vi "main.vi"() -> ()   [LabVIEW 2019]
uses:
  Globals.vi
  <vilib>/Utility/config.llb/NI_LVConfig.lvlib
panel:
  in  "sorted":bool
  in  "compare":bool
  in  "Presets":bool
  in  "Data":u16(ring) items=["cumulative cases", "new cases per day", "cumulative deaths", "new deaths per day"]
  in  "Compare with":u16(ring) items=["Don't compare", "Afghanistan", "Albania", "Algeria", "Andorra", "Angola", "Antigua and Barbuda", "Argentina", "Armenia", "Australia, Australian Capital Territory", "Australia, New South Wales", "Australia, Northern Territory", "Australia, Queensland", "Australia, South Australia", "Australia, Tasmania", "Australia, Victoria", "Australia, Western Australia", "Austria", "Azerbaijan", "Bahamas", "Bahrain", "Bangladesh", "Barbados", "Belarus", "Belgium", "Benin", "Bhutan", "Bolivia", "Bosnia and Herzegovina", "Brazil", "Brunei", "Bulgaria", "Burkina Faso", "Cabo Verde", "Cambodia", "Cameroon", "Canada, Alberta", "Canada, British Columbia", "Canada, Grand Princess", "Canada, Manitoba", "Canada, New Brunswick", "Canada, Newfoundland and Labrador", "Canada, Nova Scotia", "Canada, Ontario", "Canada, Prince Edward Island", "Canada, Quebec", "Canada, Saskatchewan", "Central African Republic", "Chad", "Chile", "China, Anhui", "China, Beijing", "China, Chongqing", "China, Fujian", "China, Gansu", "China, Guangdong", "China, Guangxi", "China, Guizhou", "China, Hainan", "China, Hebei", "China, Heilongjiang", "China, Henan", "China, Hong Kong", "China, Hubei", "China, Hunan", "China, Inner Mongolia", "China, Jiangsu", "China, Jiangxi", "China, Jilin", "China, Liaoning", "China, Macau", "China, Ningxia", "China, Qinghai", "China, Shaanxi", "China, Shandong", "China, Shanghai", "China, Shanxi", "China, Sichuan", "China, Tianjin", "China, Tibet", "China, Xinjiang", "China, Yunnan", "China, Zhejiang", "Colombia", "Congo (Brazzaville)", "Congo (Kinshasa)", "Costa Rica", "Cote d'Ivoire", "Croatia", "Diamond Princess", "Cuba", "Cyprus", "Czechia", "Denmark, Faroe Islands", "Denmark, Greenland", "Denmark", "Djibouti", "Dominican Republic", "Ecuador", "Egypt", "El Salvador", "Equatorial Guinea", "Eritrea", "Estonia", "Eswatini", "Ethiopia", "Fiji", "Finland", "France, French Guiana", "France, French Polynesia", "France, Guadeloupe", "France, Mayotte", "France, New Caledonia", "France, Reunion", "France, Saint Barthelemy", "France, St Martin", "France, Martinique", "France", "Gabon", "Gambia", "Georgia", "Germany", "Ghana", "Greece", "Guatemala", "Guinea", "Guyana", "Haiti", "Holy See", "Honduras", "Hungary", "Iceland", "India", "Indonesia", "Iran", "Iraq", "Ireland", "Israel", "Italy", "Jamaica", "Japan", "Jordan", "Kazakhstan", "Kenya", "Korea South", "Kuwait", "Kyrgyzstan", "Latvia", "Lebanon", "Liberia", "Liechtenstein", "Lithuania", "Luxembourg", "Madagascar", "Malaysia", "Maldives", "Malta", "Mauritania", "Mauritius", "Mexico", "Moldova", "Monaco", "Mongolia", "Montenegro", "Morocco", "Namibia", "Nepal", "Netherlands, Aruba", "Netherlands, Curacao", "Netherlands, Sint Maarten", "Netherlands", "New Zealand", "Nicaragua", "Niger", "Nigeria", "North Macedonia", "Norway", "Oman", "Pakistan", "Panama", "Papua New Guinea", "Paraguay", "Peru", "Philippines", "Poland", "Portugal", "Qatar", "Romania", "Russia", "Rwanda", "Saint Lucia", "Saint Vincent and the Grenadines", "San Marino", "Saudi Arabia", "Senegal", "Serbia", "Seychelles", "Singapore", "Slovakia", "Slovenia", "Somalia", "South Africa", "Spain", "Sri Lanka", "Sudan", "Suriname", "Sweden", "Switzerland", "Taiwan*", "Tanzania", "Thailand", "Togo", "Trinidad and Tobago", "Tunisia", "Turkey", "Uganda", "Ukraine", "United Arab Emirates", "United Kingdom, Bermuda", "United Kingdom, Cayman Islands", "United Kingdom, Channel Islands", "United Kingdom, Gibraltar", "United Kingdom, Isle of Man", "United Kingdom, Montserrat", "United Kingdom", "Uruguay", "US", "Uzbekistan", "Venezuela", "Vietnam", "Zambia", "Zimbabwe", "Canada, Diamond Princess", "Dominica", "Grenada", "Mozambique", "Syria", "Timor-Leste", "Belize", "Laos", "Libya", "West Bank and Gaza", "Guinea-Bissau", "Mali", "Saint Kitts and Nevis", "Canada, Northwest Territories", "Canada, Yukon", "Kosovo", "Burma", "United Kingdom, Anguilla", "United Kingdom, British Virgin Islands", "United Kingdom, Turks and Caicos Islands", "MS Zaandam", "Botswana", "Burundi", "Sierra Leone", "Netherlands, \"Bonaire Sint Eustatius and Saba\"", "Malawi", "United Kingdom, Falkland Islands (Malvinas)", "France, Saint Pierre and Miquelon", "South Sudan", "Western Sahara", "Sao Tome and Principe", "Yemen", "Comoros", "Tajikistan", "Lesotho", "Australia", "Western Europe", "Latin America", "Africa", "China", "US and Canada", "US - Northeast", "US - Midwest", "US - South", "US - West", "Scandinavia (excl Sweden)", "Global", "South Asia", "South East Asia", "East Asia", "Eastern Europe and Russia", "Middle East", "Central Asia", "American Samoa", "Guam", "Northern Mariana Islands", "Puerto Rico", "Virgin Islands", "Alabama", "Alaska", "Arizona", "Arkansas", "California", "Colorado", "Connecticut", "Delaware", "Florida", "Georgia", "Hawaii", "Idaho", "Illinois", "Indiana", "Iowa", "Kansas", "Kentucky", "Louisiana", "Maine", "Maryland", "Massachusetts", "Michigan", "Minnesota", "Mississippi", "Missouri", "Montana", "Nebraska", "Nevada", "New Hampshire", "New Jersey", "New Mexico", "New York", "North Carolina", "North Dakota", "Ohio", "Oklahoma", "Oregon", "Pennsylvania", "Rhode Island", "South Carolina", "South Dakota", "Tennessee", "Texas", "Utah", "Vermont", "Virginia", "Washington", "West Virginia", "Wisconsin", "Wyoming", "SA, EC", "SA, FS", "SA, GP", "SA, KZN", "SA, LP", "SA, MP", "SA, NC", "SA, NW", "SA, WC"]
  in  "Country":u16(ring) items=["Afghanistan", "Albania", "Algeria", "Andorra", "Angola", "Antigua and Barbuda", "Argentina", "Armenia", "Australia, Australian Capital Territory", "Australia, New South Wales", "Australia, Northern Territory", "Australia, Queensland", "Australia, South Australia", "Australia, Tasmania", "Australia, Victoria", "Australia, Western Australia", "Austria", "Azerbaijan", "Bahamas", "Bahrain", "Bangladesh", "Barbados", "Belarus", "Belgium", "Benin", "Bhutan", "Bolivia", "Bosnia and Herzegovina", "Brazil", "Brunei", "Bulgaria", "Burkina Faso", "Cabo Verde", "Cambodia", "Cameroon", "Canada, Alberta", "Canada, British Columbia", "Canada, Grand Princess", "Canada, Manitoba", "Canada, New Brunswick", "Canada, Newfoundland and Labrador", "Canada, Nova Scotia", "Canada, Ontario", "Canada, Prince Edward Island", "Canada, Quebec", "Canada, Saskatchewan", "Central African Republic", "Chad", "Chile", "China, Anhui", "China, Beijing", "China, Chongqing", "China, Fujian", "China, Gansu", "China, Guangdong", "China, Guangxi", "China, Guizhou", "China, Hainan", "China, Hebei", "China, Heilongjiang", "China, Henan", "China, Hong Kong", "China, Hubei", "China, Hunan", "China, Inner Mongolia", "China, Jiangsu", "China, Jiangxi", "China, Jilin", "China, Liaoning", "China, Macau", "China, Ningxia", "China, Qinghai", "China, Shaanxi", "China, Shandong", "China, Shanghai", "China, Shanxi", "China, Sichuan", "China, Tianjin", "China, Tibet", "China, Xinjiang", "China, Yunnan", "China, Zhejiang", "Colombia", "Congo (Brazzaville)", "Congo (Kinshasa)", "Costa Rica", "Cote d'Ivoire", "Croatia", "Diamond Princess", "Cuba", "Cyprus", "Czechia", "Denmark, Faroe Islands", "Denmark, Greenland", "Denmark", "Djibouti", "Dominican Republic", "Ecuador", "Egypt", "El Salvador", "Equatorial Guinea", "Eritrea", "Estonia", "Eswatini", "Ethiopia", "Fiji", "Finland", "France, French Guiana", "France, French Polynesia", "France, Guadeloupe", "France, Mayotte", "France, New Caledonia", "France, Reunion", "France, Saint Barthelemy", "France, St Martin", "France, Martinique", "France", "Gabon", "Gambia", "Georgia", "Germany", "Ghana", "Greece", "Guatemala", "Guinea", "Guyana", "Haiti", "Holy See", "Honduras", "Hungary", "Iceland", "India", "Indonesia", "Iran", "Iraq", "Ireland", "Israel", "Italy", "Jamaica", "Japan", "Jordan", "Kazakhstan", "Kenya", "Korea South", "Kuwait", "Kyrgyzstan", "Latvia", "Lebanon", "Liberia", "Liechtenstein", "Lithuania", "Luxembourg", "Madagascar", "Malaysia", "Maldives", "Malta", "Mauritania", "Mauritius", "Mexico", "Moldova", "Monaco", "Mongolia", "Montenegro", "Morocco", "Namibia", "Nepal", "Netherlands, Aruba", "Netherlands, Curacao", "Netherlands, Sint Maarten", "Netherlands", "New Zealand", "Nicaragua", "Niger", "Nigeria", "North Macedonia", "Norway", "Oman", "Pakistan", "Panama", "Papua New Guinea", "Paraguay", "Peru", "Philippines", "Poland", "Portugal", "Qatar", "Romania", "Russia", "Rwanda", "Saint Lucia", "Saint Vincent and the Grenadines", "San Marino", "Saudi Arabia", "Senegal", "Serbia", "Seychelles", "Singapore", "Slovakia", "Slovenia", "Somalia", "South Africa", "Spain", "Sri Lanka", "Sudan", "Suriname", "Sweden", "Switzerland", "Taiwan*", "Tanzania", "Thailand", "Togo", "Trinidad and Tobago", "Tunisia", "Turkey", "Uganda", "Ukraine", "United Arab Emirates", "United Kingdom, Bermuda", "United Kingdom, Cayman Islands", "United Kingdom, Channel Islands", "United Kingdom, Gibraltar", "United Kingdom, Isle of Man", "United Kingdom, Montserrat", "United Kingdom", "Uruguay", "US", "Uzbekistan", "Venezuela", "Vietnam", "Zambia", "Zimbabwe", "Canada, Diamond Princess", "Dominica", "Grenada", "Mozambique", "Syria", "Timor-Leste", "Belize", "Laos", "Libya", "West Bank and Gaza", "Guinea-Bissau", "Mali", "Saint Kitts and Nevis", "Canada, Northwest Territories", "Canada, Yukon", "Kosovo", "Burma", "United Kingdom, Anguilla", "United Kingdom, British Virgin Islands", "United Kingdom, Turks and Caicos Islands", "MS Zaandam", "Botswana", "Burundi", "Sierra Leone", "Netherlands, \"Bonaire Sint Eustatius and Saba\"", "Malawi", "United Kingdom, Falkland Islands (Malvinas)", "France, Saint Pierre and Miquelon", "South Sudan", "Western Sahara", "Sao Tome and Principe", "Yemen", "Comoros", "Tajikistan", "Lesotho", "Australia", "Western Europe", "Latin America", "Africa", "China", "US and Canada", "US - Northeast", "US - Midwest", "US - South", "US - West", "Scandinavia (excl Sweden)", "Global", "South Asia", "South East Asia", "East Asia", "Eastern Europe and Russia", "Middle East", "Central Asia", "American Samoa", "Guam", "Northern Mariana Islands", "Puerto Rico", "Virgin Islands", "Alabama", "Alaska", "Arizona", "Arkansas", "California", "Colorado", "Connecticut", "Delaware", "Florida", "Georgia", "Hawaii", "Idaho", "Illinois", "Indiana", "Iowa", "Kansas", "Kentucky", "Louisiana", "Maine", "Maryland", "Massachusetts", "Michigan", "Minnesota", "Mississippi", "Missouri", "Montana", "Nebraska", "Nevada", "New Hampshire", "New Jersey", "New Mexico", "New York", "North Carolina", "North Dakota", "Ohio", "Oklahoma", "Oregon", "Pennsylvania", "Rhode Island", "South Carolina", "South Dakota", "Tennessee", "Texas", "Utah", "Vermont", "Virginia", "Washington", "West Virginia", "Wisconsin", "Wyoming", "SA, EC", "SA, FS", "SA, GP", "SA, KZN", "SA, LP", "SA, MP", "SA, NC", "SA, NW", "SA, WC"]
  out "Version":u32
  in  "abs or rel":enum32{"Absolute", "Relative"}(tab)
  out "XY Graph":cluster{timestamp[], "deaths":dbl[]}[](graph)
  out "relative graph":cluster{"days":i32[], "deaths":dbl[]}[](graph)
  in  "calculate":bool
  in  "Days":u16=7
  in  "Moving average":bool
  in  "Y-axis normalised":bool
  in  "Y-axis absolute":bool caption="Y-axis"
  in  "Curve 2":enum16{"Exponential", "Logarithm", "No curve"}(ring)
  in  "Curve 1":enum16{"Exponential", "Logarithm", "No curve"}(ring)
  in  "X-axis relative":bool
  in  "X-axis absolute":bool caption="X-axis"
  in  "Curve fit cursors":bool
  in  "Curve fit all data":bool
  in  "Logarithmic":bool
  in  "threshold cases":u32=1
  in  "stop":bool
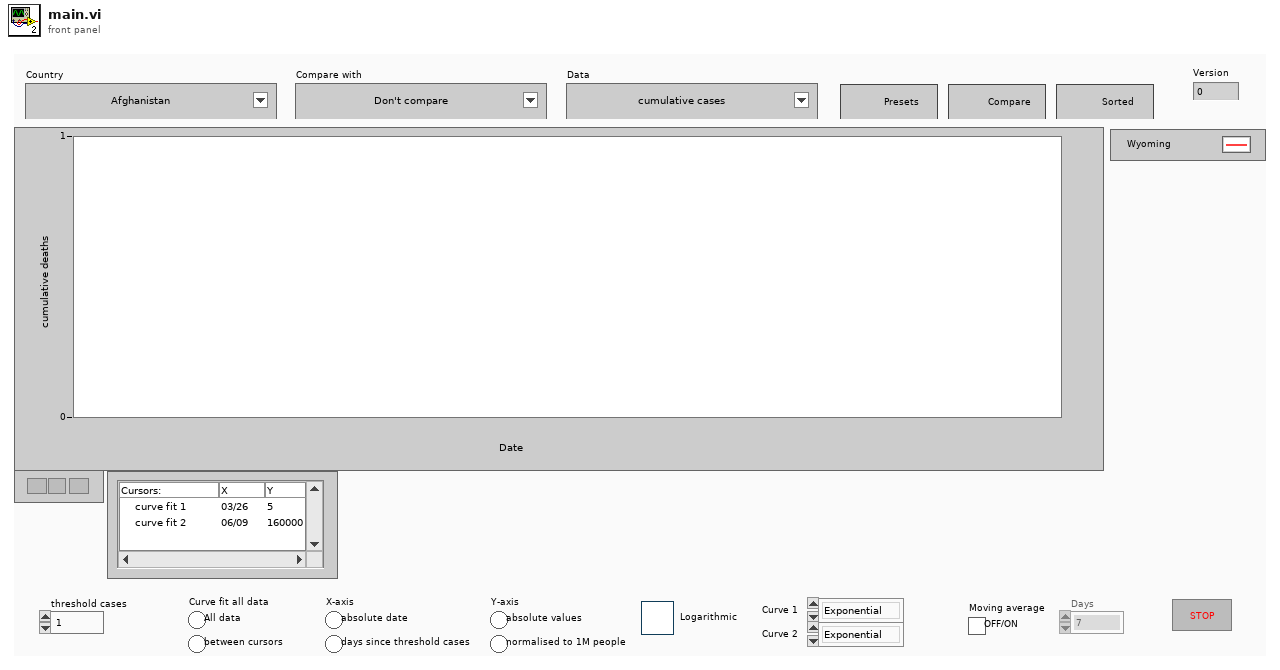
[diagram p1: front panel]
types:
  T1 = enum8{"Enabled", "Disabled", "Disabled and Grayed Out"}
  T2 = cluster{"country 1":cluster{"amplitude":dbl, "damping":dbl, "offset":dbl, "new cases per day":i32[], "days":i32[], "cumulative cases":i32[], "first case date":timestamp, "deaths":i32[], "new deaths per day":i32[]}, "country 2":cluster{"amplitude":dbl, "damping":dbl, "offset":dbl, "new cases per day":i32[], "days":i32[], "cumulative cases":i32[], "deaths":i32[], "first case date":timestamp, "new deaths per day":i32[]}, "Update plot names":refnum<user-event>}
  T3 = cluster{"cumulative deaths":i32[][], "deaths per day":i32[][], "case per day":i32[][], "cumulative cases":i32[][]}
  T4 = typedef "NI_LVConfig.lvlib/Config Data RefNum.ctl" = refnum<k1>
  T5 = cluster{"days":i32[], "new deaths per day":i32[]}
  T6 = cluster{"Country 1 index":i32, "Country 2 index":i32, "countries":string[], "Data":u16, "Curve fit all data":bool, "Curve 1 type":enum16{"Exponential", "Logarithm", "No curve"}, "Curve 2 type":enum16{"Exponential", "Logarithm", "No curve"}, "absolute?":bool, "cursor 1 ":dbl, "cursor 2 ":dbl, "threshold cases":u32}
  T7 = typedef "LVCursorListTypeDef.ctl" = cluster{"Name":string, "Color":u32, "Style":u8, "Point Style":u8, "Name Visible":bool, "Allow Drag":bool, "Cursor Mode":u32, "Plot":i32, "Index":i32, "Position":cluster{"X":dbl, "Y":dbl}, "X Scale":u32, "Y Scale":u32, "Watch Plots":i32[], "Watch All Plots":bool, "Plot Area":i32, "Label Offset":cluster{"X":dbl, "Y":dbl}}[]
  T8 = cluster{"Name":string, "Color":u32, "Style":u8, "Point Style":u8, "Name Visible":bool, "Allow Drag":bool, "Cursor Mode":u32, "Plot":i32, "Index":i32, "Position":cluster{"X":dbl, "Y":dbl}, "X Scale":u32, "Y Scale":u32, "Watch Plots":i32[], "Watch All Plots":bool, "Plot Area":i32, "Label Offset":cluster{"X":dbl, "Y":dbl}}
  T9 = cluster{"days":i32[], "moving average array":dbl[]}
  T10 = cluster{"days":i32[], "moving average array":dbl[]}[]
  T11 = cluster{timestamp[], "moving average array":dbl[]}
  T12 = cluster{timestamp[], "moving average array":dbl[]}[]
  T13 = cluster{"Name":string, "Color":u32, "Style":u8, "Point Style":u8, "Name Visible":bool, "Allow Drag":bool, "Cursor Mode":u32, "Plot":i32, "Index":i32, "Position":cluster{"X":dbl, "Y":dbl}, "X Scale":u32, "Y Scale":u32, "Watch Plots":i32[], "Watch All Plots":bool, "Plot Area":i32, "Label Offset":cluster{"X":dbl, "Y":dbl}}[]
  T14 = typedef "LVRangeTypeDef.ctl" = cluster{"Minimum":dbl, "Maximum":dbl, "Increment":dbl, "Minor Increment":dbl, "Start":dbl}
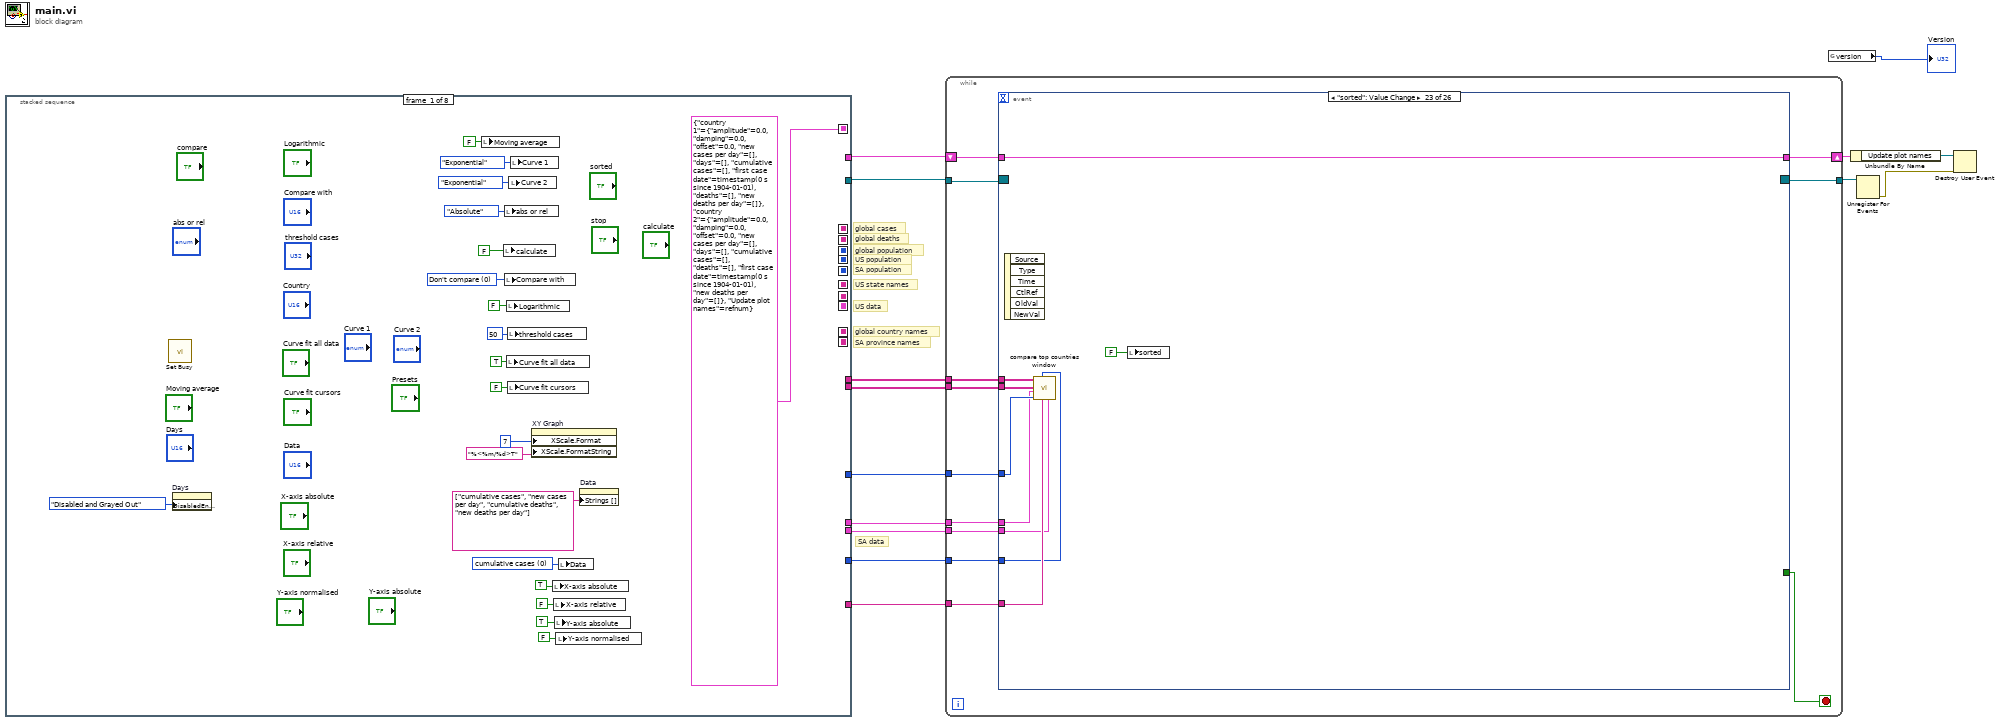
[diagram p0: block diagram]
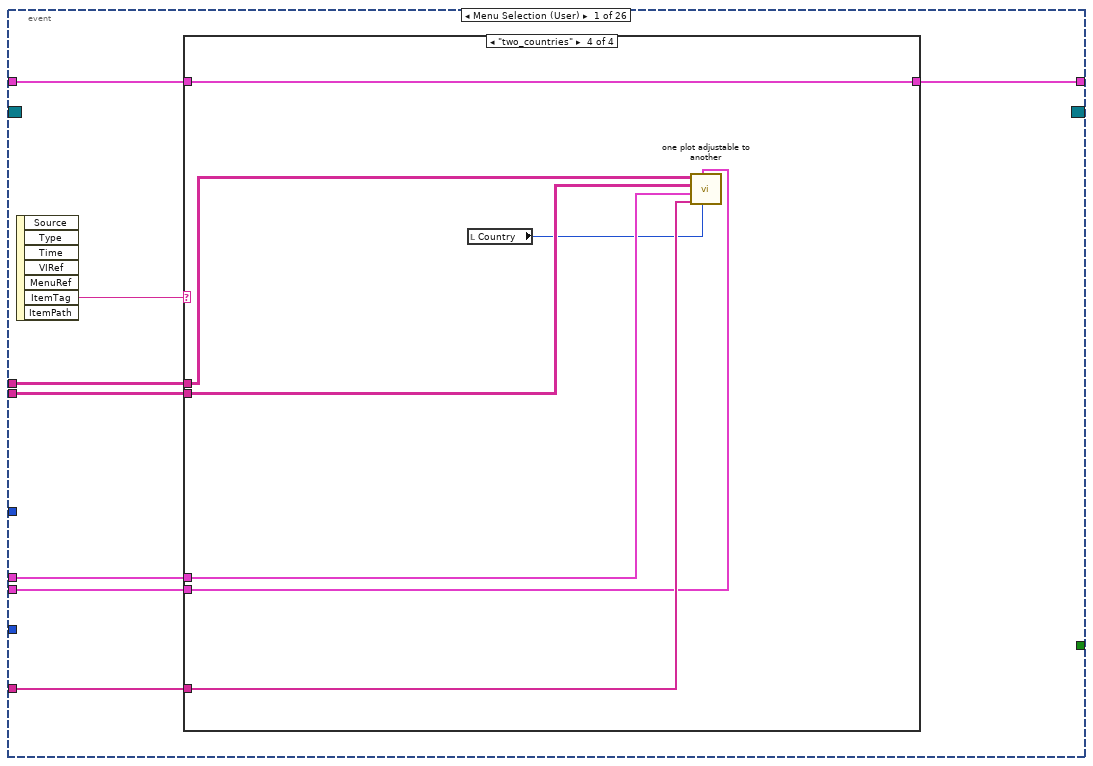
[diagram p2: hidden frame]
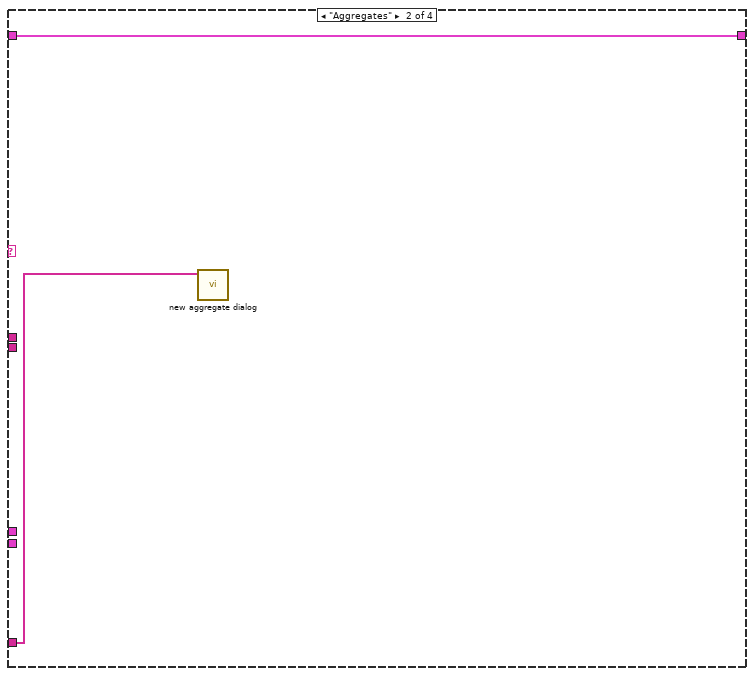
[diagram p4: hidden frame]
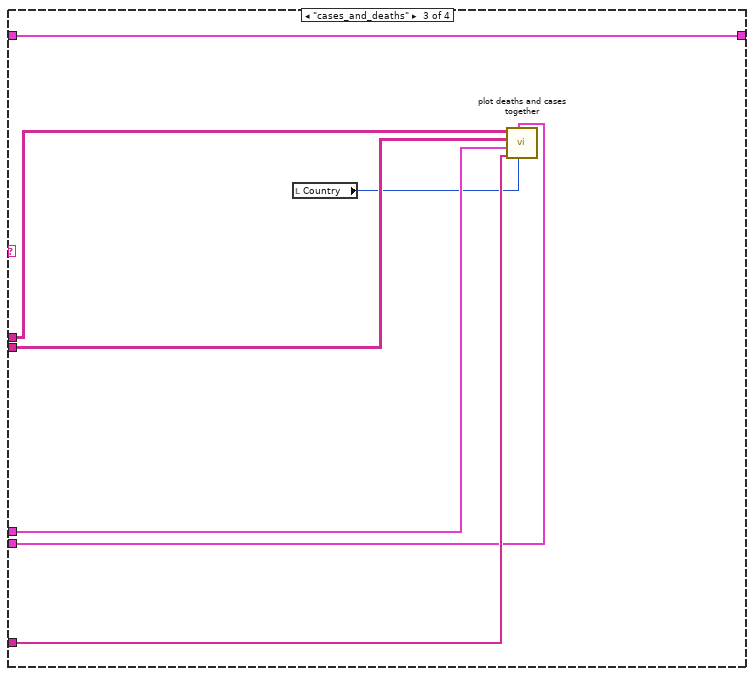
[diagram p5: hidden frame]
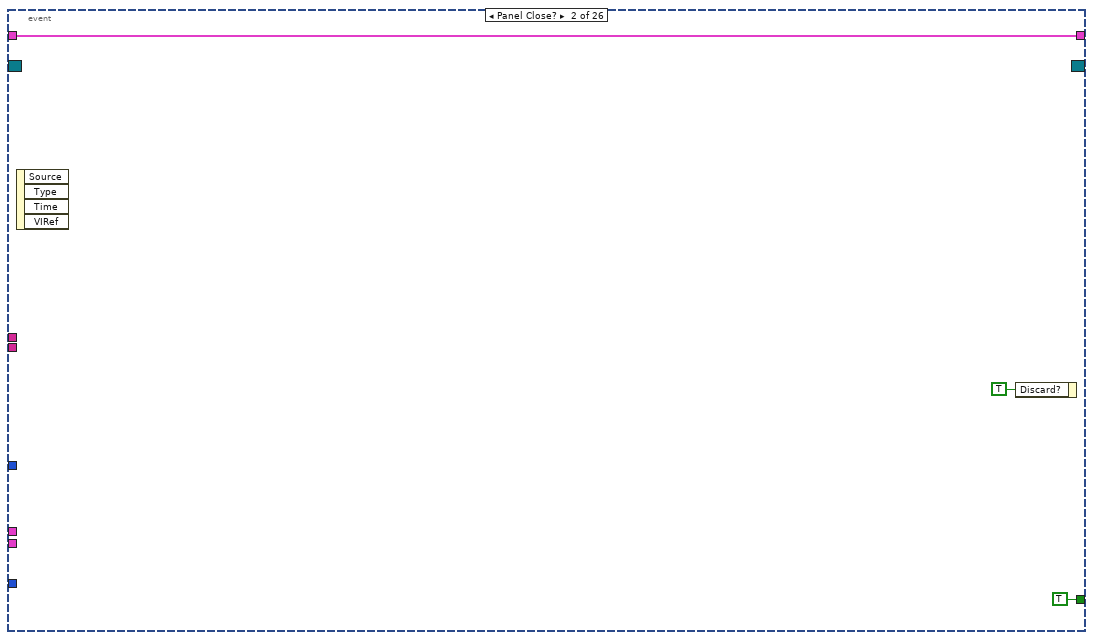
[diagram p6: hidden frame]
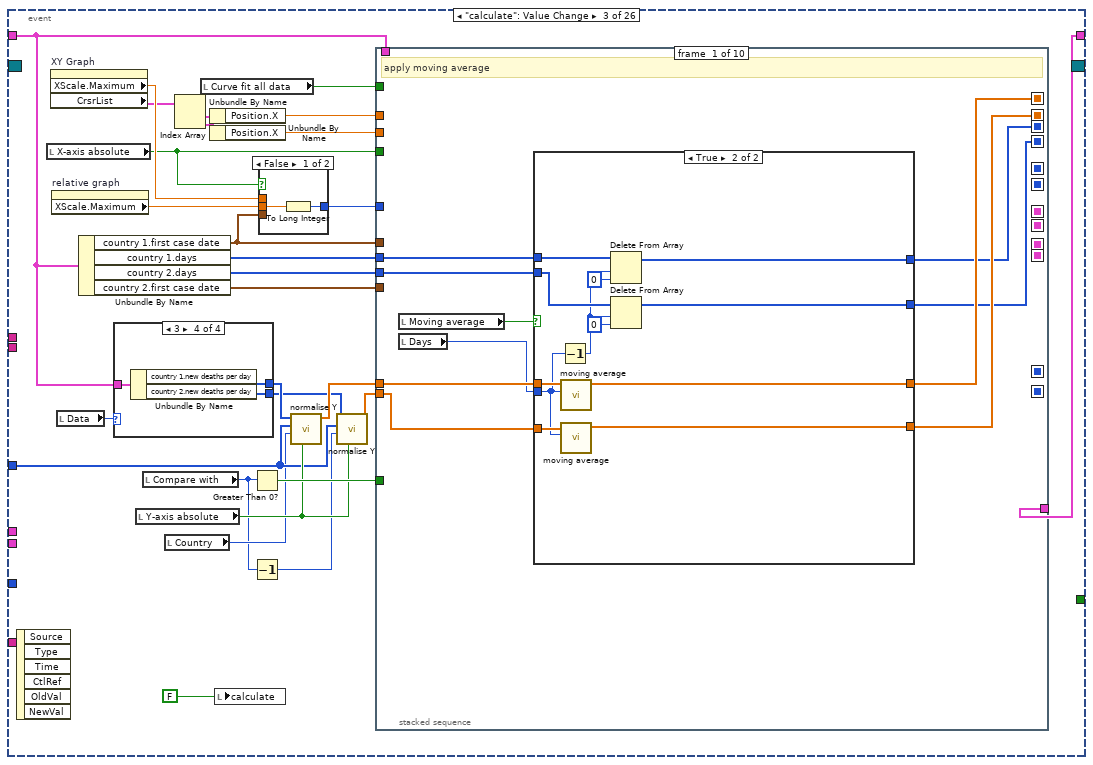
[diagram p7: hidden frame]
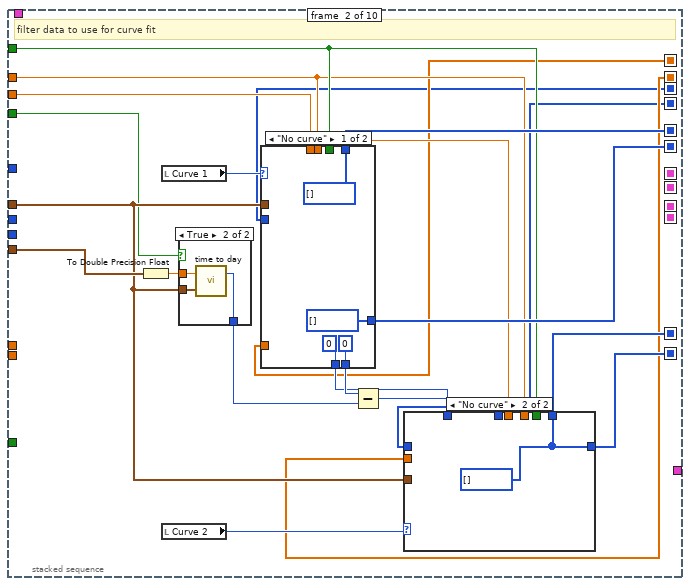
[diagram p9: hidden frame]
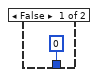
[diagram p10: hidden frame]
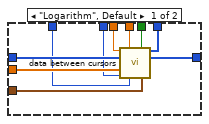
[diagram p11: hidden frame]
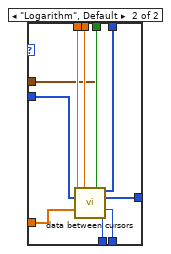
[diagram p12: hidden frame]
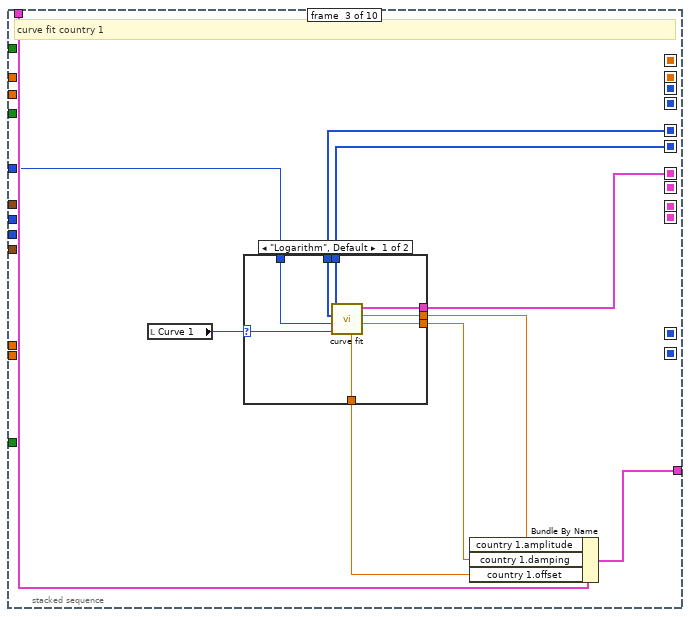
[diagram p13: hidden frame]
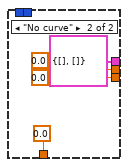
[diagram p14: hidden frame]
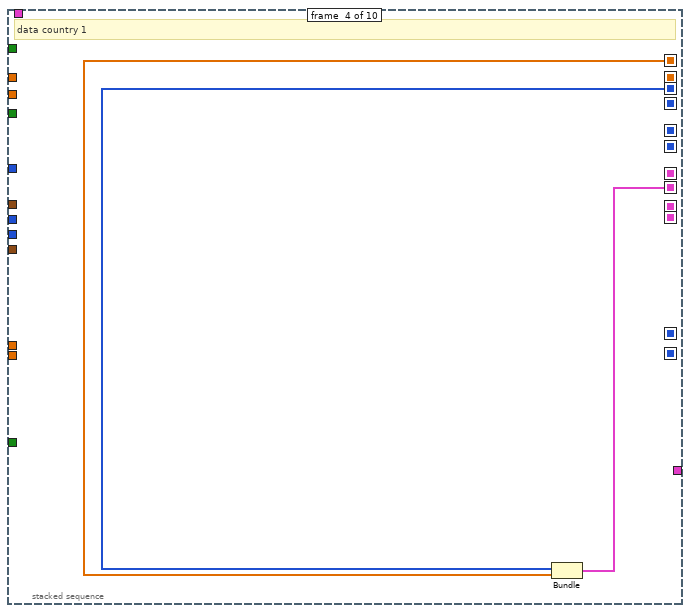
[diagram p15: hidden frame]
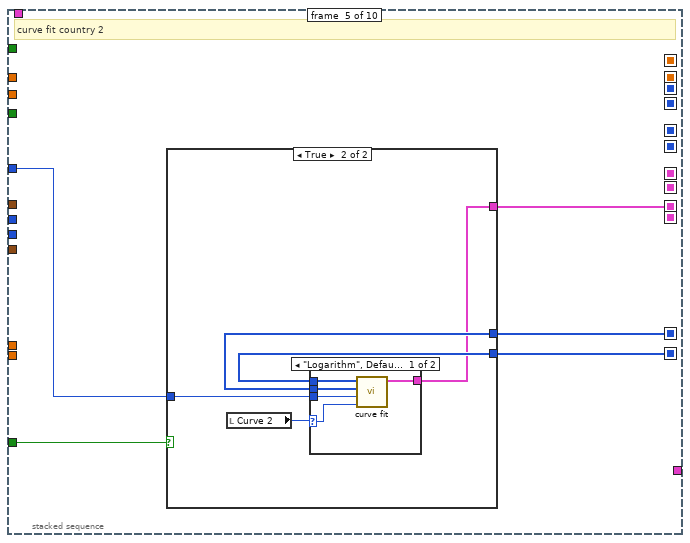
[diagram p16: hidden frame]
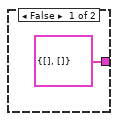
[diagram p17: hidden frame]
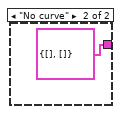
[diagram p18: hidden frame]
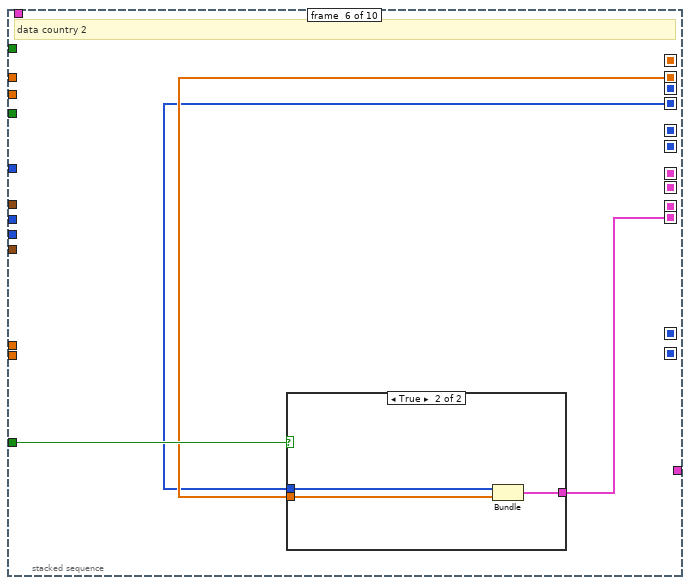
[diagram p19: hidden frame]
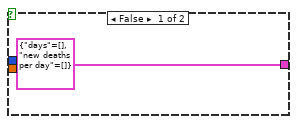
[diagram p20: hidden frame]
diagram:
  # "SA data"
  # "SA province names"
  # "global country names"
  # "US data"
  # "global deaths"
  # "global cases"
  # "US state names"
  # "SA population"
  # "US population"
  # "global population"
  n1 = stacked-sequence {
    seq-local: [T2 {"country 1"={"amplitude"=0.0, "damping"=0.0, "offset"=0.0, "new cases per day"=[], "days"=[], "cumulative cases"=[], "first case date"=timestamp(0 s since 1904-01-01), "deaths"=[], "new deaths per day"=[]}, "country 2"={"amplitude"=0.0, "damping"=0.0, "offset"=0.0, "new cases per day"=[], "days"=[], "cumulative cases"=[], "deaths"=[], "first case date"=timestamp(0 s since 1904-01-01), "new deaths per day"=[]}, "Update plot names"=refnum} _ _ _ _ _ _ _] -> [_ _ _ _ _ _ _ w160]
    seq-local: [_ w45 _ _ _ _ _ _] -> [_ _ _ w69 w96 _ _ _]
    seq-local: [_ _ w56 _ _ _ _ _] -> [_ _ _ _ w108 _ _ _]
    seq-local: [_ _ w55 _ _ _ _ _] -> [_ _ _ _ w105 _ _ _]
    seq-local: [_ _ w49 _ _ _ _ _] -> [_ _ _ _ w104 _ _ _]
    seq-local: [_ _ w48 _ _ _ _ _] -> [_ _ _ _ w98 w131 _ _]
    seq-local: [_ _ _ _ w101 _ _ _] -> [_ _ _ _ _ w133 _ _]
    seq-local: [_ _ w50 _ _ _ _ _] -> [_ _ _ _ w100 _ _ _]
    seq-local: [_ _ _ w68 _ _ _ _] -> [_ _ _ _ w99 _ _ _]
    seq-local: [_ _ w54 _ _ _ _ _] -> [_ _ _ _ w91 _ _ _]
    seq-local: [_ _ w52 _ _ _ _ _] -> [_ _ _ _ _ w129 _ _]
    tunnel: [_ _ _ _ w101 _ _ _] -> w14
    tunnel: [_ _ _ _ _ _ _ w159] -> w13
    tunnel: [_ _ _ _ w106 _ _ _] -> w12
    tunnel: [_ _ _ _ w102 _ _ _] -> w11
    tunnel: [_ _ w50 _ _ _ _ _] -> w10
    tunnel: [_ _ _ _ _ w132 _ _] -> w9
    tunnel: [_ _ _ _ _ _ _ w162] -> w8
    tunnel: [_ _ _ _ w95 _ _ _] -> w3
    tunnel: [_ _ w51 _ _ _ _ _] -> w2
    frame #0 {
      w25 = u16 0 items=["cumulative cases", "new cases per day"] ("Data")
      w33 = u16 0 items=["Don't compare", "Afghanistan", "Albania", "Algeria", "Andorra", "Angola", "Antigua and Barbuda", "Argentina", "Armenia", "Australia, Australian Capital Territory", "Australia, New South Wales", "Australia, Northern Territory", "Australia, Queensland", "Australia, South Australia", "Australia, Tasmania", "Australia, Victoria", "Australia, Western Australia", "Austria", "Azerbaijan", "Bahamas", "Bahrain", "Bangladesh", "Barbados", "Belarus", "Belgium", "Benin", "Bhutan", "Bolivia", "Bosnia and Herzegovina", "Brazil", "Brunei", "Bulgaria", "Burkina Faso", "Cabo Verde", "Cambodia", "Cameroon", "Canada, Alberta", "Canada, British Columbia", "Canada, Grand Princess", "Canada, Manitoba", "Canada, New Brunswick", "Canada, Newfoundland and Labrador", "Canada, Nova Scotia", "Canada, Ontario", "Canada, Prince Edward Island", "Canada, Quebec", "Canada, Saskatchewan", "Central African Republic", "Chad", "Chile", "China, Anhui", "China, Beijing", "China, Chongqing", "China, Fujian", "China, Gansu", "China, Guangdong", "China, Guangxi", "China, Guizhou", "China, Hainan", "China, Hebei", "China, Heilongjiang", "China, Henan", "China, Hong Kong", "China, Hubei", "China, Hunan", "China, Inner Mongolia", "China, Jiangsu", "China, Jiangxi", "China, Jilin", "China, Liaoning", "China, Macau", "China, Ningxia", "China, Qinghai", "China, Shaanxi", "China, Shandong", "China, Shanghai", "China, Shanxi", "China, Sichuan", "China, Tianjin", "China, Tibet", "China, Xinjiang", "China, Yunnan", "China, Zhejiang", "Colombia", "Congo (Brazzaville)", "Congo (Kinshasa)", "Costa Rica", "Cote d'Ivoire", "Croatia", "Diamond Princess", "Cuba", "Cyprus", "Czechia", "Denmark, Faroe Islands", "Denmark, Greenland", "Denmark", "Djibouti", "Dominican Republic", "Ecuador", "Egypt", "El Salvador", "Equatorial Guinea", "Eritrea", "Estonia", "Eswatini", "Ethiopia", "Fiji", "Finland", "France, French Guiana", "France, French Polynesia", "France, Guadeloupe", "France, Mayotte", "France, New Caledonia", "France, Reunion", "France, Saint Barthelemy", "France, St Martin", "France, Martinique", "France", "Gabon", "Gambia", "Georgia", "Germany", "Ghana", "Greece", "Guatemala", "Guinea", "Guyana", "Haiti", "Holy See", "Honduras", "Hungary", "Iceland", "India", "Indonesia", "Iran", "Iraq", "Ireland", "Israel", "Italy", "Jamaica", "Japan", "Jordan", "Kazakhstan", "Kenya", "\"Korea", "Kuwait", "Kyrgyzstan", "Latvia", "Lebanon", "Liberia", "Liechtenstein", "Lithuania", "Luxembourg", "Madagascar", "Malaysia", "Maldives", "Malta", "Mauritania", "Mauritius", "Mexico", "Moldova", "Monaco", "Mongolia", "Montenegro", "Morocco", "Namibia", "Nepal", "Netherlands, Aruba", "Netherlands, Curacao", "Netherlands, Sint Maarten", "Netherlands", "New Zealand", "Nicaragua", "Niger", "Nigeria", "North Macedonia", "Norway", "Oman", "Pakistan", "Panama", "Papua New Guinea", "Paraguay", "Peru", "Philippines", "Poland", "Portugal", "Qatar", "Romania", "Russia", "Rwanda", "Saint Lucia", "Saint Vincent and the Grenadines", "San Marino", "Saudi Arabia", "Senegal", "Serbia", "Seychelles", "Singapore", "Slovakia", "Slovenia", "Somalia", "South Africa", "Spain", "Sri Lanka", "Sudan", "Suriname", "Sweden", "Switzerland", "Taiwan*", "Tanzania", "Thailand", "Togo", "Trinidad and Tobago", "Tunisia", "Turkey", "Uganda", "Ukraine", "United Arab Emirates", "United Kingdom, Bermuda", "United Kingdom, Cayman Islands", "United Kingdom, Channel Islands", "United Kingdom, Gibraltar", "United Kingdom, Isle of Man", "United Kingdom, Montserrat", "United Kingdom", "Uruguay", "US", "Uzbekistan", "Venezuela", "Vietnam", "Zambia", "Zimbabwe", "Canada, Diamond Princess", "Dominica", "Grenada", "Mozambique", "Syria", "Timor-Leste", "Belize", "Canada, Recovered", "Laos", "Libya", "The West Bank and Gaza"] ("Compare with")
      n2 = call <vilib>:"Set Busy.vi"() -> ()  [unwired: 10 in, 2 out]
      n3 = property on="Days" class="DigNum (strict)"("DisabledEnum"=T1."Disabled and Grayed Out" ("Disabled")) -> ()  [unwired: 2 in, 2 out]
      n4 = local write "Moving average"(FALSE ("Moving average")) -> ()
      n5 = local write "calculate"(FALSE ("Blank Button")) -> ()
      n6 = local write "abs or rel"(enum32{"Absolute", "Relative"}."Absolute" ("abs or rel")) -> ()
      n7 = local write "Compare with"(w33) -> ()
      n8 = local write "Logarithmic"(FALSE ("Logarithmic")) -> ()
      n9 = local write "Curve fit all data"(TRUE ("Curve fit all data")) -> ()
      n10 = local write "threshold cases"(u32 50 ("threshold cases")) -> ()
      n11 = local write "Curve fit cursors"(FALSE ("Curve fit cursors")) -> ()
      n12 = local write "Curve 2"(enum16{"Exponential", "Logarithm"}."Exponential" ("Curve 2")) -> ()
      n13 = local write "Curve 1"(enum16{"Exponential", "Logarithm"}."Exponential" ("Curve 1")) -> ()
      n14 = property on="XY Graph" class="XYGraph (strict)"("XScale.Format"=u8 7 ("X Scale.Display Format:Format"), "XScale.FormatString"="%<%m/%d>T" ("X Scale.Format String")) -> ()  [unwired: 2 in, 2 out]
      n15 = local write "X-axis absolute"(TRUE ("X-axis absolute")) -> ()
      n16 = local write "X-axis relative"(FALSE ("X-axis relative")) -> ()
      n17 = local write "Y-axis absolute"(TRUE ("Y-axis absolute")) -> ()
      n18 = local write "Y-axis normalised"(FALSE ("Y-axis normalised")) -> ()
      n19 = local write "Data"(w25) -> ()
      n20 = property on="Data" class="Ring (strict)"("Strings []"=string[] ["cumulative cases", "new cases per day", "cumulative deaths", "new deaths per day"]) -> ()  [unwired: 2 in, 2 out]
    }
    frame #1 {
      # "get global cases in 2D string matrix"
      n21 = global read "Globals.vi" "Global cases URL"() -> (w36:string)
      n22 = call "download file.vi"("URL"=w36, "Error message"="Could not download global cases") -> ("downloaded file"=w35:string)  [unwired: 8 in, 1 out]
      n23 = Search and Replace String(replace all?=TRUE ("replace all? (F)"), input string=w35, search string=", ", replace string=" " ("replace string (\"\")")) -> (result string=w38:string)  [unwired: 4 in, 3 out]
      n24 = Spreadsheet String To Array(delimiter (Tab)=",", format string="%s", spreadsheet string=w38, array type (2D Dbl)=string[][] []) -> (array=w45:string[][])
    }
    frame #2 {
      # "get global deaths in 2D string matrix, get population data and US data and SA data"
      n25 = global read "Globals.vi" "Global deaths URL"() -> (w47:string)
      n26 = call "download file.vi"("URL"=w47, "Error message"="Could not download Global deaths CSV" ("message")) -> ("downloaded file"=w58:string)  [unwired: 8 in, 1 out]
      n27 = Search and Replace String(replace all?=TRUE ("replace all? (F)"), input string=w58, search string=", ", replace string=" " ("replace string (\"\")")) -> (result string=w57:string)  [unwired: 4 in, 3 out]
      n28 = Spreadsheet String To Array(delimiter (Tab)=",", format string="%s", spreadsheet string=w57, array type (2D Dbl)=string[][] []) -> (array=w56:string[][])
      n29 = call "create population index.vi"("deaths global csv array"=w56) -> ("Populations"=w55:i32[])  [unwired: 9 in, 1 out]
      n30 = call "get all US data.vi"() -> ("populations"=w49:i32[], "cases countries"=w48:string[], "US data"=w50:T3)  [unwired: 9 in]
      n31 = call "get SA province data.vi"() -> ("populations"=w54:i32[], "SA province names"=w53:string[], "SA data"=w51:T3)  [unwired: 9 in]
      n32 = for {
        tunnel: w53 -> [w65] mode=indexing
        tunnel: [w67] -> w52 mode=indexing
        n33 = Concatenate Strings("SA, " ("string"), w65) -> (w67:string)
      }
    }
    frame #3 {
      n34 = Index Array(array=w69, index (col)=1 ("disabled index (col)")) -> (element=w77:string[])  [unwired: 1 in]
      n35 = Index Array(array=w69, index (col)=0 ("disabled index (col)")) -> (element=w75:string[])  [unwired: 1 in]
      n36 = Array Subset(array=w77, index=1) -> (w76:string[])  [unwired: 1 in]
      n37 = Array Subset(array=w75, index=1) -> (w74:string[])  [unwired: 1 in]
      n38 = for {
        tunnel: w76 -> [w79] mode=indexing
        tunnel: w74 -> [w83] mode=indexing
        tunnel: [w84] -> w68 mode=indexing
        n39 = Empty String/Path?(string/path=w83) -> (empty?=w85:bool)
        n40 = Search and Replace String(replace all?=TRUE ("replace all? (F)"), input string=w79, search string="\"", replace string="" ("replace string (\"\")")) -> (result string=w78:string)  [unwired: 4 in, 3 out]
        n41 = case shown="False" w85 {
          tunnel: w78 -> [w89 w90]
          tunnel: [w86 w90] -> w84
          tunnel: w83 -> [w87 _]
          frame False {
            n42 = Concatenate Strings(w89, ", " ("string"), w87) -> (w86:string)
          }
          frame True {
          }
        }
      }
    }
    frame #4 {
      # "load aggregates"
      n43 = call "get aggregate names.vi"() -> ("section names"=w112:string[], "Refnum out"=w111:T4)  [unwired: 10 in]
      n44 = Array Size(array=w96) -> (size(s)=w93:i32[])
      n45 = Build Array (concatenate)(w99, w98) -> (w97:string[])
      n46 = Index Array(array=w93) -> (element=w92:i32)  [unwired: 1 in]
      n47 = Decrement(x=w92) -> (x-1=w94:i32)
      n48 = for {
        tunnel: w112 -> [w118] mode=indexing
        shift-right: [w127] -> w110
        shift-left: w111 -> [w128]
        tunnel: w96 -> [w126]
        tunnel: w108 -> [w125]
        tunnel: w105 -> [w124]
        tunnel: w104 -> [w122]
        tunnel: [w121] -> w109 mode=indexing
        tunnel: [w120] -> w107 mode=indexing
        tunnel: [w119] -> w103 mode=indexing
        tunnel: w100 -> [w117]
        tunnel: w97 -> [w116]
        tunnel: w94 -> [w114]
        tunnel: [w113] -> w95 mode=indexing
        i -> [w115]
        n49 = call "get countries in aggregate.vi"("countries"=w116, "aggregate name"=w118, "Refnum in"=w128) -> ("country indexes"=w123:i32[], "Refnum out"=w127:T4)  [unwired: 7 in]
        n50 = call "create aggregate stats.vi"("US data"=w117, "Aggregate name"=w118, "country indexes of aggregate"=w123, "populations US"=w122, "Populations global"=w124, "global deaths"=w125, "global cases"=w126) -> ("population"=w119:i64, "deaths array array"=w120:string[], "cases array"=w121:string[])  [unwired: 2 in]
        n51 = Add(x=w114, y=w115) -> (x+y=w113:i32)
      }
      n52 = call <vilib>:"Close Config Data.vi"("refnum"=w110) -> ()  [unwired: 9 in, 2 out]
      n53 = Build Array (concatenate)(w96, w109) -> (w101:string[][])
      n54 = Build Array (concatenate)(w108, w107) -> (w106:string[][])
      n55 = Build Array (concatenate)(w105, w103, w104, w91) -> (w102:i64[])
    }
    frame #5 {
      n56 = Index Array(array=w133, index (col)=1 ("disabled index (col)")) -> (element=w144:string[])  [unwired: 1 in]
      n57 = Index Array(array=w133, index (col)=0 ("disabled index (col)")) -> (element=w142:string[])  [unwired: 1 in]
      n58 = Array Subset(array=w144, index=1) -> (w143:string[])  [unwired: 1 in]
      n59 = Array Subset(array=w142, index=1) -> (w141:string[])  [unwired: 1 in]
      n60 = for {
        tunnel: w143 -> [w146] mode=indexing
        tunnel: w141 -> [w150] mode=indexing
        tunnel: [w151] -> w130 mode=indexing
        n61 = Empty String/Path?(string/path=w150) -> (empty?=w152:bool)
        n62 = Search and Replace String(replace all?=TRUE ("replace all? (F)"), input string=w146, search string="\"", replace string="" ("replace string (\"\")")) -> (result string=w145:string)  [unwired: 4 in, 3 out]
        n63 = case shown="False" w152 {
          tunnel: w145 -> [w156 w157]
          tunnel: [w153 w157] -> w151
          tunnel: w150 -> [w154 _]
          frame False {
            n64 = Concatenate Strings(w156, ", " ("string"), w154) -> (w153:string)
          }
          frame True {
          }
        }
      }
      n65 = Build Array (concatenate)(w130, w131, w129) -> (w132:string[])
      n66 = Build Array (concatenate)("Don't compare", w132) -> (w140:string[])
      n67 = property on="Compare with" class="Ring (strict)"("Strings []"=w140) -> ()  [unwired: 2 in, 2 out]
      n68 = property on="Country" class="Ring (strict)"("Strings []"=w132, "Val(Sgnl)"=u16 200 ("Value (Signaling)")) -> ()  [unwired: 2 in, 2 out]
    }
    frame #6 {
      n69 = call <vilib>:"Unset Busy.vi"() -> ()  [unwired: 11 in, 1 out]
    }
    frame #7 {
      w161 = TRUE  # Update plot names
      n70 = Create User Event(user event datatype=w161) -> (user event=w158:refnum<user-event>)  [unwired: 1 in, 1 out]
      n71 = register-events(w158) -> (reference out=w162:refnum<event-registration>)  [unwired: 2 in, 1 out]
      n72 = Bundle By Name(cluster=w160, "Update plot names"=w158) -> (w159:T2)
    }
  }
  n73 = while {
    tunnel: w14 -> [w173]
    shift-right: [w171] -> w7
    shift-left: w13 -> [w172]
    tunnel: w12 -> [w170]
    tunnel: w11 -> [w169]
    tunnel: w10 -> [w168]
    tunnel: w9 -> [w167]
    tunnel: w8 -> [w166]
    tunnel: [w165] -> w5
    tunnel: w3 -> [w164]
    tunnel: w2 -> [w163]
    stop <- w174 stop-if-true
    n74 = event shown="[22] \"sorted\": Value Change" {
      selector: w166 -> [_ _ _ _ _ _ _ _ _ _ _ _ _ _ _ _ _ _ _ _ _ _ _ _ _ _]
      dyn-events: [_ _ _ _ _ _ _ _ _ _ _ _ _ _ _ _ _ _ _ _ _ _ _ _ _ _] -> w165
      timeout: _ -> [_ _ _ _ _ _ _ _ _ _ _ _ _ _ _ _ _ _ _ _ _ _ _ _ _ _]
      tunnel: [_ TRUE _ _ TRUE _ _ _ _ _ _ _ _ _ _ _ _ _ _ _ _ _ _ FALSE _ _] -> w174
      tunnel: w173 -> [w178 _ _ _ _ w594 w638 _ _ _ _ _ _ _ _ _ _ _ _ _ w756 w883 w892 _ _ _]
      tunnel: w172 -> [w182 w202 w225 w574 w578 w583 w624 w655 w658 w661 w665 w684 w700 w714 w728 w735 w742 w745 w748 w751 w758 w884 w893 w900 w902 w919]
      tunnel: [w181 w202 w229 w574 w578 w604 w634 w655 w658 w661 w665 w684 w700 w714 w728 w735 w742 w745 w748 w751 w757 w884 w893 w900 w902 w919] -> w171
      tunnel: w170 -> [w177 _ _ _ _ w593 w631 _ _ _ _ _ _ _ _ _ _ _ _ _ w755 w882 w891 _ _ _]
      tunnel: w169 -> [_ _ w206 _ _ _ _ _ _ _ _ _ _ _ _ _ _ _ _ _ _ w880 w889 _ _ _]
      tunnel: w168 -> [w176 _ _ _ _ w584 w627 _ _ _ _ _ _ _ _ _ _ _ _ _ w754 w879 w888 _ _ _]
      tunnel: w167 -> [w179 _ _ _ _ _ _ _ _ _ _ _ _ _ _ _ _ _ _ _ _ w878 w887 _ _ _]
      tunnel: w164 -> [_ _ _ _ _ _ _ _ _ _ _ _ _ _ _ _ _ _ _ _ _ w877 w886 _ _ _]
      tunnel: w163 -> [w175 _ _ _ _ w580 w623 _ _ _ _ _ _ _ _ _ _ _ _ _ w753 w876 w885 _ _ _]
      event Menu Selection (User) {
        n75 = event-data() -> ("ItemTag"=w180:string)  [unwired: 1 in, 6 out]
        n76 = case shown="\"two_countries\"" w180 {
          tunnel: w182 -> [w183 w185 w192 w199]
          tunnel: [w183 w185 w192 w199] -> w181
          tunnel: w179 -> [_ w184 w188 w195]
          tunnel: w178 -> [_ _ w191 w198]
          tunnel: w177 -> [_ _ w190 w197]
          tunnel: w176 -> [_ _ w189 w196]
          tunnel: w175 -> [_ _ w186 w193]
          frame "False", Default {
          }
          frame "Aggregates" {
            n77 = call "new aggregate dialog.vi"("Countries"=w184) -> ()  [unwired: 11 in]
          }
          frame "cases_and_deaths" {
            n78 = local read "Country"() -> (w187:u16)
            n79 = call "plot deaths and cases together.vi"("country index"=w187, "SA data"=w186, "Countries (in)"=w188, "US data"=w189, "deaths CSV"=w190, "cases CSV"=w191) -> ()  [unwired: 6 in]
          }
          frame "two_countries" {
            n80 = local read "Country"() -> (w194:u16)
            n81 = call "one plot adjustable to another.vi"("country index"=w194, "SA data"=w193, "Countries (in)"=w195, "US data"=w196, "deaths CSV"=w197, "cases CSV"=w198) -> ()  [unwired: 6 in]
          }
        }
      }
      event Panel Close? {
        n82 = event-data() -> ()  [unwired: 1 in, 4 out]
        n83 = event-data("Discard?"=TRUE) -> ()  [unwired: 1 in, 1 out]
      }
      event "calculate": Value Change {
        n84 = event-data() -> ()  [unwired: 1 in, 6 out]
        n85 = local read "X-axis absolute"() -> (w215:bool)
        n86 = property on="XY Graph" class="XYGraph (strict)"() -> ("XScale.Maximum"=w227:dbl, "CrsrList"=w219:T7)  [unwired: 2 in, 2 out]
        n87 = property on="relative graph" class="XYGraph (strict)"() -> ("XScale.Maximum"=w213:dbl)  [unwired: 2 in, 2 out]
        n88 = local read "Data"() -> (w226:u16)
        n89 = Unbundle By Name(w225) -> ("country 1.first case date"=w223:timestamp, "country 1.days"=w224:i32[], "country 2.days"=w222:i32[], "country 2.first case date"=w214:timestamp)
        n90 = case shown="3" w226 {
          tunnel: [w562 w565 w568 w571] -> w211
          tunnel: w225 -> [w563 w566 w569 w572]
          tunnel: [w561 w564 w567 w570] -> w209
          frame 0, Default {
            n91 = Unbundle By Name(w563) -> ("country 1.cumulative cases"=w562:i32[], "country 2.cumulative cases"=w561:i32[])
          }
          frame 1 {
            n92 = Unbundle By Name(w566) -> ("country 1.new cases per day"=w565:i32[], "country 2.new cases per day"=w564:i32[])
          }
          frame 2 {
            n93 = Unbundle By Name(w569) -> ("country 1.deaths"=w568:i32[], "country 2.deaths"=w567:i32[])
          }
          frame 3 {
            n94 = Unbundle By Name(w572) -> ("country 1.new deaths per day"=w571:i32[], "country 2.new deaths per day"=w570:i32[])
          }
        }
        n95 = local read "Y-axis absolute"() -> (w207:bool)
        n96 = local read "Compare with"() -> (w204:u16)
        n97 = local read "Country"() -> (w205:u16)
        n98 = Index Array(array=w219) -> (element #1=w221:T8, element #2=w220:T8)  [unwired: 2 in]
        n99 = local read "Curve fit all data"() -> (w216:bool)
        n100 = Unbundle By Name(w221) -> ("Position.X"=w218:dbl)
        n101 = Unbundle By Name(w220) -> ("Position.X"=w217:dbl)
        n102 = local write "calculate"(FALSE ("Blank Button")) -> ()
        n103 = Greater Than 0?(x=w204) -> (x > 0?=w212:bool)
        n104 = Decrement(x=w204) -> (x-1=w203:u16)
        n105 = case shown="False" w215 {
          tunnel: [w557 w560] -> w228
          tunnel: w227 -> [_ w559]
          tunnel: w223 -> [_ w558]
          tunnel: w213 -> [w556 _]
          frame False {
            n106 = To Long Integer(number=w556) -> (32bit integer=w557:i32)
          }
          frame True {
            n107 = call "time to day.vi"("time offset"=w558, "time in seconds"=w559) -> ("nearest day"=w560:i32)  [unwired: 1 out]
          }
        }
        n108 = call "normalise Y.vi"("Y-axis absolute"=w207, "Country index"=w205, "Populations"=w206, "Y in"=w211) -> ("Y out"=w210:dbl[])  [unwired: 7 in]
        n109 = call "normalise Y.vi"("Y-axis absolute"=w207, "Country index"=w203, "Populations"=w206, "Y in"=w209) -> ("Y out"=w208:dbl[])  [unwired: 7 in]
        n110 = stacked-sequence {
          seq-local: [_ _ w316 _ _ _ _ _ _ _] -> [_ _ _ _ _ _ w364 w412 _ _]
          seq-local: [_ _ _ _ w333 _ _ _ _ _] -> [_ _ _ _ _ _ w362 w410 _ _]
          seq-local: [_ w277 _ _ _ _ _ _ _ _] -> [_ _ w314 _ _ _ _ _ _ _]
          seq-local: [_ w276 _ _ _ _ _ _ _ _] -> [_ _ w315 _ _ _ _ _ _ _]
          seq-local: [_ w270 _ _ _ _ _ _ _ _] -> [_ _ _ _ w335 _ _ _ _ _]
          seq-local: [_ w269 _ _ _ _ _ _ _ _] -> [_ _ _ _ w334 _ _ _ _ _]
          seq-local: [_ _ _ w331 _ _ _ _ _ _] -> [_ _ _ _ _ _ w363 w411 _ _]
          seq-local: [_ _ _ _ _ w352 _ _ _ _] -> [_ _ _ _ _ _ w361 w409 _ _]
          seq-local: [w236 _ _ _ _ _ _ _ _ _] -> [_ w260 _ w330 _ _ _ _ _ _]
          seq-local: [w235 _ _ _ _ _ _ _ _ _] -> [_ w259 _ _ _ w350 _ _ _ _]
          seq-local: [w232 _ _ _ _ _ _ _ _ _] -> [_ w258 _ w329 _ _ _ _ _ _]
          seq-local: [w231 _ _ _ _ _ _ _ _ _] -> [_ w257 _ _ _ w349 _ _ _ _]
          tunnel: w228 -> [_ _ w308 _ w336 _ _ _ _ _]
          tunnel: w208 -> [w237 _ _ _ _ _ _ _ _ _]
          tunnel: w222 -> [w233 _ _ _ _ _ _ _ _ _]
          tunnel: w224 -> [w234 _ _ _ _ _ _ _ _ _]
          tunnel: w210 -> [w240 _ _ _ _ _ _ _ _ _]
          tunnel: w225 -> [_ _ w313 _ _ _ _ _ _ _]
          tunnel: [_ _ w312 _ _ _ _ _ _ _] -> w229
          tunnel: w223 -> [_ w265 _ _ _ _ _ w408 _ _]
          tunnel: w218 -> [_ w274 _ _ _ _ _ _ _ _]
          tunnel: w217 -> [_ w273 _ _ _ _ _ _ _ _]
          tunnel: w216 -> [_ w275 _ _ _ _ _ _ _ _]
          tunnel: w215 -> [_ w261 _ _ _ _ _ _ _ _]
          tunnel: w214 -> [_ w268 _ _ _ _ _ w407 _ _]
          tunnel: w212 -> [_ _ _ _ w332 w351 w359 w395 w471 _]
          frame #0 {
            # "apply moving average"
            n111 = local read "Moving average"() -> (w238:bool)
            n112 = local read "Days"() -> (w239:u16)
            n113 = case shown="True" w238 {
              tunnel: w240 -> [w244 w256]
              tunnel: w239 -> [_ w251]
              tunnel: [w244 w255] -> w236
              tunnel: w237 -> [w243 w254]
              tunnel: [w243 w253] -> w235
              tunnel: w234 -> [w242 w252]
              tunnel: w233 -> [w241 w250]
              tunnel: [w242 w246] -> w232
              tunnel: [w241 w245] -> w231
              frame False {
              }
              frame True {
                n114 = Decrement(x=w251) -> (x-1=w249:u16)
                n115 = call "moving average.vi"("average over x points"=w251, "Array"=w256) -> ("moving average array"=w255:dbl[])  [unwired: 8 in, 1 out]
                n116 = call "moving average.vi"("average over x points"=w251, "Array"=w254) -> ("moving average array"=w253:dbl[])  [unwired: 8 in, 1 out]
                n117 = Delete From Array(array=w252, length=w249, index=0) -> (array with subset deleted=w246:i32[])  [unwired: 1 out]
                n118 = Delete From Array(array=w250, length=w249, index=0) -> (array with subset deleted=w245:i32[])  [unwired: 1 out]
              }
            }
          }
          frame #1 {
            # "filter data to use for curve fit"
            n119 = To Double Precision Float(number=w268) -> (double precision float=w264:dbl)
            n120 = local read "Curve 1"() -> (w263:enum16{"Exponential", "Logarithm", "No curve"})
            n121 = local read "Curve 2"() -> (w262:enum16{"Exponential", "Logarithm", "No curve"})
            n122 = case shown="True" w261 {
              tunnel: [0 ("nearest day") w281] -> w266
              tunnel: w265 -> [_ w280]
              tunnel: w264 -> [_ w279]
              frame False {
              }
              frame True {
                n123 = call "time to day.vi"("time offset"=w280, "time in seconds"=w279) -> ("nearest day"=w281:i32)  [unwired: 1 out]
              }
            }
            n124 = case shown="\"No curve\"" w263 {
              tunnel: w258 -> [_ w306]
              tunnel: w260 -> [_ w305]
              tunnel: [i32[] [] ("X out") w304] -> w277
              tunnel: [i32[] [] ("Y out") w303] -> w276
              tunnel: w275 -> [_ w302]
              tunnel: w274 -> [_ w301]
              tunnel: w273 -> [_ w300]
              tunnel: [0 ("index start out") w299] -> w272
              tunnel: [0 ("array length out") w298] -> w271
              tunnel: w265 -> [_ w297]
              frame "No curve" {
              }
              frame "Logarithm", Default {
                n125 = call "data between cursors.vi"("cursor 1 X"=w300, "cursor 2 X"=w301, "Curve fit all data"=w302, "X in"=w306, "Y in"=w305, "first case date"=w297) -> ("X out"=w304:i32[], "Y out"=w303:i32[], "index start out"=w299:i32, "array length out"=w298:i32)  [unwired: 6 in]
              }
            }
            n126 = Subtract(x=w272, y=w266) -> (x-y=w267:i32)
            n127 = case shown="\"No curve\"" w262 {
              tunnel: w257 -> [w291 _]
              tunnel: w259 -> [w290 _]
              tunnel: w275 -> [w289 _]
              tunnel: w274 -> [w288 _]
              tunnel: w273 -> [w287 _]
              tunnel: w271 -> [w286 _]
              tunnel: [w285 w292] -> w270
              tunnel: [w284 w292] -> w269
              tunnel: w267 -> [w283 _]
              tunnel: w265 -> [w282 _]
              frame "Logarithm", Default {
                n128 = call "data between cursors.vi"("cursor 1 X"=w287, "cursor 2 X"=w288, "Curve fit all data"=w289, "X in"=w291, "Y in"=w290, "index start in"=w283, "array length in"=w286, "first case date"=w282) -> ("X out"=w285:i32[], "Y out"=w284:i32[])  [unwired: 4 in, 2 out]
              }
              frame "No curve" {
                w292 = i32[] [] ("Y out")
              }
            }
          }
          frame #2 {
            # "curve fit country 1"
            n129 = local read "Curve 1"() -> (w307:enum16{"Exponential", "Logarithm", "No curve"})
            n130 = case shown="\"Logarithm\", Default" w307 {
              selector: w307 -> [w317 _]
              tunnel: [w324 cluster{i32[], dbl[]} {[], []} ("Cluster")] -> w316
              tunnel: w315 -> [w323 _]
              tunnel: w314 -> [w322 _]
              tunnel: [w321 0.0 ("amplitude")] -> w311
              tunnel: [w320 0.0 ("damping")] -> w310
              tunnel: [w319 0.0 ("offset")] -> w309
              tunnel: w308 -> [w318 _]
              frame "Logarithm", Default {
                n131 = call "curve fit.vi"("Curve fit"=w317, "day"=w318, "X"=w322, "Y"=w323) -> ("damping"=w320:dbl, "amplitude"=w321:dbl, "Cluster"=w324:cluster{i32[], dbl[]}, "offset"=w319:dbl)  [unwired: 4 in]
              }
              frame "No curve" {
              }
            }
            n132 = Bundle By Name(cluster=w313, "country 1.amplitude"=w311, "country 1.damping"=w310, "country 1.offset"=w309) -> (w312:T2)
          }
          frame #3 {
            # "data country 1"
            n133 = Bundle("days"=w329, "moving average array"=w330) -> (w331:T9)  [unwired: 1 in]
          }
          frame #4 {
            # "curve fit country 2"
            n134 = case shown="True" w332 {
              tunnel: w336 -> [_ w342]
              tunnel: w335 -> [_ w341]
              tunnel: w334 -> [_ w340]
              tunnel: [cluster{i32[], dbl[]} {[], []} ("Cluster") w339] -> w333
              frame False {
              }
              frame True {
                n135 = local read "Curve 2"() -> (w338:enum16{"Exponential", "Logarithm", "No curve"})
                n136 = case shown="\"Logarithm\", Default" w338 {
                  selector: w338 -> [w343 _]
                  tunnel: w342 -> [w347 _]
                  tunnel: w341 -> [w346 _]
                  tunnel: w340 -> [w345 _]
                  tunnel: [w344 cluster{i32[], dbl[]} {[], []} ("Cluster")] -> w339
                  frame "Logarithm", Default {
                    n137 = call "curve fit.vi"("Curve fit"=w343, "day"=w347, "X"=w346, "Y"=w345) -> ("Cluster"=w344:cluster{i32[], dbl[]})  [unwired: 4 in, 3 out]
                  }
                  frame "No curve" {
                  }
                }
              }
            }
          }
          frame #5 {
            # "data country 2"
            n138 = case shown="True" w351 {
              tunnel: w350 -> [_ w354]
              tunnel: [T5 {"days"=[], "new deaths per day"=[]} w356] -> w352
              tunnel: w349 -> [_ w355]
              frame False {
              }
              frame True {
                n139 = Bundle("days"=w355, "moving average array"=w354) -> (w356:T9)  [unwired: 1 in]
              }
            }
          }
          frame #6 {
            # "adjust legend rows and x-axis and update graph"
            n140 = local read "Curve 2"() -> (w357:enum16{"Exponential", "Logarithm", "No curve"})
            n141 = local read "Curve 1"() -> (w358:enum16{"Exponential", "Logarithm", "No curve"})
            n142 = case shown="True" w359 {
              tunnel: w364 -> [w367 w382]
              tunnel: w363 -> [w366 w381]
              tunnel: w362 -> [_ w379]
              tunnel: w361 -> [_ w378]
              tunnel: [w368 w375] -> w360
              tunnel: w358 -> [w365 w380]
              tunnel: w357 -> [_ w374]
              frame False {
                n143 = case shown="\"Logarithm\", Default" w365 {
                  tunnel: [w370 w373] -> w368
                  tunnel: w367 -> [_ w372]
                  tunnel: w366 -> [w369 w371]
                  frame "No curve" {
                    n144 = Build Array(w369) -> (w370:T10)
                  }
                  frame "Logarithm", Default {
                    n145 = Build Array(w372, w371) -> (w373:T10)
                  }
                }
              }
              frame True {
                n146 = case shown="\"No curve\"" w380 {
                  tunnel: w382 -> [w390 _]
                  tunnel: w381 -> [w389 w392]
                  tunnel: [w388 w391] -> w377
                  frame "Logarithm", Default {
                    n147 = Build Array(w390, w389) -> (w388:T10)
                  }
                  frame "No curve" {
                    n148 = Build Array(w392) -> (w391:T10)
                  }
                }
                n149 = case shown="\"No curve\"" w374 {
                  tunnel: w379 -> [w385 _]
                  tunnel: [w384 w386] -> w376
                  tunnel: w378 -> [w383 w387]
                  frame "Logarithm", Default {
                    n150 = Build Array(w385, w383) -> (w384:T10)
                  }
                  frame "No curve" {
                    n151 = Build Array(w387) -> (w386:T10)
                  }
                }
                n152 = Build Array (concatenate)(w377, w376) -> (w375:T10)
              }
            }
            "relative graph" <- w360
          }
          frame #7 {
            # "adjust legend rows and x-axis and update graph"
            n153 = case shown="False" w395 {
              tunnel: w410 -> [_ w452]
              tunnel: w409 -> [_ w451]
              tunnel: w407 -> [_ w450]
              tunnel: [w441 w449] -> w398
              tunnel: [w441 w448] -> w397
              frame False {
                w441 = cluster{timestamp[], dbl[]} {[], []}
              }
              frame True {
                n154 = Unbundle(w452) -> (w445:i32[], w447:dbl[])
                n155 = Unbundle(w451) -> ("days"=w444:i32[], "moving average array"=w446:dbl[])
                n156 = for {
                  tunnel: w445 -> [w458] mode=indexing
                  tunnel: w450 -> [w457]
                  tunnel: [w456] -> w442 mode=indexing
                  n157 = call "day to time.vi"("Time offset"=w457, "day"=w458) -> ("day in absolute time"=w456:timestamp)  [unwired: 1 out]
                }
                n158 = for {
                  tunnel: w444 -> [w455] mode=indexing
                  tunnel: w450 -> [w454]
                  tunnel: [w453] -> w443 mode=indexing
                  n159 = call "day to time.vi"("Time offset"=w454, "day"=w455) -> ("day in absolute time"=w453:timestamp)  [unwired: 1 out]
                }
                n160 = Bundle(w442, w447) -> (w449:cluster{timestamp[], dbl[]})  [unwired: 1 in]
                n161 = Bundle(w443, "moving average array"=w446) -> (w448:T11)  [unwired: 1 in]
              }
            }
            n162 = Unbundle(w412) -> (w406:i32[], w404:dbl[])
            n163 = Unbundle(w411) -> ("days"=w401:i32[], "moving average array"=w400:dbl[])
            n164 = for {
              tunnel: w406 -> [w464] mode=indexing
              tunnel: w408 -> [w463]
              tunnel: [w462] -> w405 mode=indexing
              n165 = call "day to time.vi"("Time offset"=w463, "day"=w464) -> ("day in absolute time"=w462:timestamp)  [unwired: 1 out]
            }
            n166 = for {
              tunnel: w401 -> [w461] mode=indexing
              tunnel: w408 -> [w460]
              tunnel: [w459] -> w402 mode=indexing
              n167 = call "day to time.vi"("Time offset"=w460, "day"=w461) -> ("day in absolute time"=w459:timestamp)  [unwired: 1 out]
            }
            n168 = Bundle(w405, w404) -> (w403:cluster{timestamp[], dbl[]})  [unwired: 1 in]
            n169 = Bundle(w402, "moving average array"=w400) -> (w399:T11)  [unwired: 1 in]
            n170 = local read "Curve 1"() -> (w394:enum16{"Exponential", "Logarithm", "No curve"})
            n171 = local read "Curve 2"() -> (w393:enum16{"Exponential", "Logarithm", "No curve"})
            n172 = case shown="False" w395 {
              tunnel: w403 -> [w416 w428]
              tunnel: w399 -> [w415 w427]
              tunnel: w398 -> [_ w426]
              tunnel: w397 -> [_ w425]
              tunnel: [w414 w422] -> w396
              tunnel: w394 -> [w413 w430]
              tunnel: w393 -> [_ w429]
              frame False {
                n173 = case shown="\"No curve\"" w413 {
                  tunnel: w416 -> [_ w421]
                  tunnel: w415 -> [w418 w420]
                  tunnel: [w417 w419] -> w414
                  frame "No curve" {
                    n174 = Build Array(w418) -> (w417:T12)
                  }
                  frame "Logarithm", Default {
                    n175 = Build Array(w421, w420) -> (w419:T12)
                  }
                }
              }
              frame True {
                n176 = case shown="\"Logarithm\", Default" w429 {
                  tunnel: w426 -> [w433 _]
                  tunnel: [w432 w434] -> w423
                  tunnel: w425 -> [w431 w435]
                  frame "Logarithm", Default {
                    n177 = Build Array(w433, w431) -> (w432:T12)
                  }
                  frame "No curve" {
                    n178 = Build Array(w435) -> (w434:T12)
                  }
                }
                n179 = case shown="\"Logarithm\", Default" w430 {
                  tunnel: w428 -> [w438 _]
                  tunnel: w427 -> [w437 w440]
                  tunnel: [w436 w439] -> w424
                  frame "Logarithm", Default {
                    n180 = Build Array(w438, w437) -> (w436:T12)
                  }
                  frame "No curve" {
                    n181 = Build Array(w440) -> (w439:T12)
                  }
                }
                n182 = Build Array (concatenate)(w424, w423) -> (w422:T12)
              }
            }
            "XY Graph" <- w396
          }
          frame #8 {
            (unwired) u32 4375295 ("Plot.Plot Color 4")
            (unwired) u32 982784 ("Plot.Plot Color 3")
            (unwired) u32 16728642 ("Plot.Plot Color 2")
            (unwired) u32 483491 ("Plot.Plot Color")
            n183 = local read "Curve 1"() -> (w470:enum16{"Exponential", "Logarithm", "No curve"})
            n184 = local read "Curve 2"() -> (w469:enum16{"Exponential", "Logarithm", "No curve"})
            n185 = case shown="True" w471 {
              tunnel: w470 -> [w481 w507]
              tunnel: w469 -> [_ w506]
              tunnel: [w480 w503] -> w468
              tunnel: [w479 w500] -> w466
              tunnel: [w478 w498] -> w465
              frame False {
                n186 = case shown="\"No curve\"" w481 {
                  tunnel: [w488 w495] -> w480
                  tunnel: [w485 w493] -> w479
                  tunnel: [w484 w491] -> w478
                  frame "Exponential", Default {
                    n187 = Build Array(u32 483491 ("Plot.Plot Color"), u32 16728642 ("Plot.Plot Color 2")) -> (w484:u32[])
                    n188 = Build Array(0, 6) -> (w485:i32[])
                    n189 = Build Array(2, 0) -> (w488:i32[])
                  }
                  frame "No curve" {
                    n190 = Build Array(u32 16728642 ("Plot.Plot Color 2")) -> (w491:u32[])
                    n191 = Build Array(u8 0 ("Plot.Plot Interpolation")) -> (w493:u8[])
                    n192 = Build Array(u8 2 ("Plot.Plot Interpolation")) -> (w495:u8[])
                  }
                }
              }
              frame True {
                n193 = case shown="\"No curve\"" w507 {
                  tunnel: [w529 w536] -> w505
                  tunnel: [w526 w534] -> w502
                  tunnel: [w523 w532] -> w499
                  frame "Exponential", Default {
                    n194 = Build Array(0, 6) -> (w526:i32[])
                    n195 = Build Array(2, 0) -> (w529:i32[])
                    n196 = Build Array(u32 483491 ("Plot.Plot Color"), u32 16728642 ("Plot.Plot Color 2")) -> (w523:u32[])
                  }
                  frame "No curve" {
                    n197 = Build Array(u32 16728642 ("Plot.Plot Color 2")) -> (w532:u32[])
                    n198 = Build Array(u8 0 ("Plot.Plot Interpolation")) -> (w534:u8[])
                    n199 = Build Array(u8 2 ("Plot.Plot Interpolation")) -> (w536:u8[])
                  }
                }
                n200 = case shown="\"No curve\"" w506 {
                  tunnel: [w515 w522] -> w504
                  tunnel: [w512 w519] -> w501
                  tunnel: [w510 w518] -> w497
                  frame "Exponential", Default {
                    n201 = Build Array(u32 982784 ("Plot.Plot Color 3"), u32 4375295 ("Plot.Plot Color 4")) -> (w510:u32[])
                    n202 = Build Array(u8 0 ("Plot.Plot Interpolation"), u8 6 ("element")) -> (w512:u8[])
                    n203 = Build Array(u8 2 ("Plot.Plot Interpolation"), u8 0 ("element")) -> (w515:u8[])
                  }
                  frame "No curve" {
                    n204 = Build Array(u32 4375295 ("Plot.Plot Color 4")) -> (w518:u32[])
                    n205 = Build Array(0) -> (w519:i32[])
                    n206 = Build Array(2) -> (w522:i32[])
                  }
                }
                n207 = Build Array (concatenate)(w499, w497) -> (w498:u32[])
                n208 = Build Array (concatenate)(w502, w501) -> (w500:i32[])
                n209 = Build Array (concatenate)(w505, w504) -> (w503:i32[])
              }
            }
            n210 = for {
              tunnel: w468 -> [w474] mode=indexing
              tunnel: w466 -> [w473] mode=indexing
              tunnel: w465 -> [w472] mode=indexing
              i -> [w477]
              n211 = property on="XY Graph" class="XYGraph (strict)"("Active Plot"=w477) -> (error out=w475:errorcluster)  [unwired: 2 in, 1 out]
              n212 = property on="relative graph" class="XYGraph (strict)"("Active Plot"=w477) -> (error out=w476:errorcluster)  [unwired: 2 in, 1 out]
              n213 = property on="relative graph" class="XYGraph (strict)"(error in=w476, "Plot.Plot Interpolation"=w474, "Plot.Point Style"=w473, "Plot.Plot Color"=w472) -> ()  [unwired: 1 in, 2 out]
              n214 = property on="XY Graph" class="XYGraph (strict)"(error in=w475, "Plot.Plot Interpolation"=w474, "Plot.Point Style"=w473, "Plot.Plot Color"=w472) -> ()  [unwired: 1 in, 2 out]
            }
            n215 = Array Size(array=w465) -> (size(s)=w467:i32)
            n216 = property on="relative graph" class="XYGraph (strict)"("LegNumRows"=w467) -> ()  [unwired: 2 in, 2 out]
            n217 = property on="XY Graph" class="XYGraph (strict)"("LegNumRows"=w467) -> ()  [unwired: 2 in, 2 out]
          }
          frame #9 {
            n218 = local read "Moving average"() -> (w542:bool)
            n219 = local read "Days"() -> (w543:u16)
            n220 = property on="Data" class="Ring (strict)"() -> ("Strings []"=w547:string[], "Value"=w546:u16)  [unwired: 2 in, 2 out]
            n221 = local read "Y-axis absolute"() -> (w545:bool)
            n222 = Index Array(array=w547, index=w546) -> (element=w550:string)
            n223 = local read "threshold cases"() -> (w538:u32)
            n224 = Not(x=w545) -> (.not. x?=w544:bool)
            n225 = Format Into String(format string=" (%d days mov avg)", w543) -> (resulting string=w549:string)  [unwired: 2 in, 1 out]
            n226 = Select(t=" per 1M", s=w544, f="") -> (s? t:f=w555:string)
            n227 = Select(t=w549, s=w542, f="") -> (s? t:f=w552:string)
            n228 = Format Into String(format string="Days since %d cases", w538) -> (resulting string=w540:string)  [unwired: 2 in, 1 out]
            n229 = Concatenate Strings(w550, w555, w552) -> (w541:string)
            n230 = property on="relative graph" class="XYGraph (strict)"("XScale.NameLbl.Text"=w540) -> ()  [unwired: 2 in, 2 out]
            n231 = property on="relative graph" class="XYGraph (strict)"("YScale.NameLbl.Text"=w541) -> ()  [unwired: 2 in, 2 out]
            n232 = property on="XY Graph" class="XYGraph (strict)"("YScale.NameLbl.Text"=w541) -> ()  [unwired: 2 in, 2 out]
          }
        }
      }
      event "Logarithmic": Value Change {
        n233 = event-data() -> ("NewVal"=w577:bool)  [unwired: 1 in, 5 out]
        n234 = Select(t=u8 1, s=w577, f=u8 0 ("Y Scale.Mapping Mode")) -> (s? t:f=w573:u8)
        n235 = property on="XY Graph" class="XYGraph (strict)"("YScale.Mapping Mode"=w573) -> ()  [unwired: 2 in, 2 out]
        n236 = property on="relative graph" class="XYGraph (strict)"("YScale.Mapping Mode"=w573) -> ()  [unwired: 2 in, 2 out]
      }
      event "stop": Value Change {
        n237 = event-data() -> ()  [unwired: 1 in, 6 out]
      }
      event "Country": Value Change {
        w596 = 0 ("day")
        n238 = event-data() -> ("NewVal"=w585:u16)  [unwired: 1 in, 5 out]
        n239 = local read "threshold cases"() -> (w592:u32)
        n240 = local read "Compare with"() -> (w619:u16)
        n241 = call "parse CSV files.vi"("threshold cases"=w592, "SA data"=w580, "US data"=w584, "deaths CSV"=w593, "country index"=w585, "cases CSV"=w594) -> ("new deaths per day"=w586:i32[], "days"=w588:i32[], "new cases per day"=w589:i32[], "first case date"=w591:timestamp, "cumulative cases"=w587:i32[], "cumulative deaths"=w590:i32[])
        n242 = Greater Than 0?(x=w619) -> (x > 0?=w620:bool)
        n243 = case shown="False" w620 {
          tunnel: w619 -> [_ w622]
          frame False {
            n244 = property on="calculate" class="Bool (strict)"("Val(Sgnl)"=TRUE ("Value (Signaling)")) -> ()  [unwired: 2 in, 2 out]
          }
          frame True {
            n245 = property on="Compare with" class="Ring (strict)"("Val(Sgnl)"=w622) -> ()  [unwired: 2 in, 2 out]
          }
        }
        n246 = property on="XY Graph" class="XYGraph (strict)"() -> ("CrsrList"=w618:T7)  [unwired: 2 in, 2 out]
        n247 = property on="relative graph" class="XYGraph (strict)"() -> ("CrsrList"=w603:T7)  [unwired: 2 in, 2 out]
        n248 = Array Size(array=w587) -> (size(s)=w597:i32)
        n249 = Index Array(array=w618) -> (element #1=w617:T8, element #2=w616:T8)  [unwired: 2 in]
        n250 = Index Array(array=w603) -> (element #1=w602:T8, element #2=w601:T8)  [unwired: 2 in]
        n251 = Unbundle By Name(w583) -> ("Update plot names"=w582:refnum<user-event>)
        n252 = Add(x=6, y=w597) -> (x+y=w595:i32)
        n253 = call "day to time.vi"("Time offset"=w591, "day"=w596) -> ("day in seconds"=w605:dbl)  [unwired: 1 out]
        n254 = call "day to time.vi"("Time offset"=w591, "day"=w597) -> ("day in seconds"=w606:dbl)  [unwired: 1 out]
        n255 = Bundle By Name(cluster=w602, "Position.X"=w596) -> (w600:T8)
        n256 = Bundle By Name(cluster=w601, "Position.X"=w597) -> (w599:T8)
        n257 = call "day to time.vi"("Time offset"=w591, "day"=w595) -> ("day in seconds"=w607:dbl)  [unwired: 1 out]
        n258 = Generate User Event(user event=w582, event data cluster=TRUE ("event data")) -> ()  [unwired: 2 in, 2 out]
        n259 = Bundle By Name(cluster=w617, "Position.X"=w605, "Allow Drag"=TRUE, "Cursor Mode"=u32 0) -> (w615:T8)
        n260 = Bundle By Name(cluster=w616, "Position.X"=w606, "Allow Drag"=TRUE, "Cursor Mode"=u32 0) -> (w614:T8)
        n261 = Build Array(w615, w614) -> (w613:T13)
        n262 = Build Array(w600, w599) -> (w598:T13)
        n263 = Bundle By Name(cluster=w583, "country 1.first case date"=w591, "country 1.days"=w588, "country 1.cumulative cases"=w587, "country 1.new cases per day"=w589, "country 1.deaths"=w590, "country 1.new deaths per day"=w586) -> (w604:T2)
        n264 = property on="XY Graph" class="XYGraph (strict)"("CrsrList"=w613, "XScale.Maximum"=w607, "XScale.Minimum"=w605) -> ()  [unwired: 2 in, 2 out]
        n265 = property on="relative graph" class="XYGraph (strict)"("CrsrList"=w598, "XScale.Minimum"=w596, "XScale.Maximum"=w595) -> ()  [unwired: 2 in, 2 out]
      }
      event "Compare with": Value Change {
        n266 = event-data() -> ("NewVal"=w636:u16)  [unwired: 1 in, 5 out]
        n267 = Greater Than 0?(x=w636) -> (x > 0?=w637:bool)
        n268 = case shown="True" w637 {
          tunnel: w638 -> [_ w647]
          tunnel: w636 -> [_ w649]
          tunnel: [w640 w653] -> w635
          tunnel: [w640 w652] -> w633
          tunnel: [w640 w651] -> w632
          tunnel: w631 -> [_ w650]
          tunnel: [w640 w648] -> w630
          tunnel: [timestamp(0 s since 1904-01-01) w646] -> w629
          tunnel: [w640 w645] -> w628
          tunnel: w627 -> [_ w643]
          tunnel: w623 -> [_ w642]
          frame False {
            w640 = i32[] []
          }
          frame True {
            n269 = Decrement(x=w649) -> (x-1=w644:u16)
            n270 = local read "threshold cases"() -> (w654:u32)
            n271 = call "parse CSV files.vi"("threshold cases"=w654, "SA data"=w642, "US data"=w643, "deaths CSV"=w650, "country index"=w644, "cases CSV"=w647) -> ("new deaths per day"=w645:i32[], "days"=w652:i32[], "new cases per day"=w653:i32[], "first case date"=w646:timestamp, "cumulative cases"=w651:i32[], "cumulative deaths"=w648:i32[])
          }
        }
        n272 = property on="calculate" class="Bool (strict)"("Val(Sgnl)"=TRUE ("Value (Signaling)")) -> ()  [unwired: 2 in, 2 out]
        n273 = Unbundle By Name(w624) -> ("Update plot names"=w626:refnum<user-event>)
        n274 = Bundle By Name(cluster=w624, "country 2.first case date"=w629, "country 2.new cases per day"=w635, "country 2.days"=w633, "country 2.cumulative cases"=w632, "country 2.deaths"=w630, "country 2.new deaths per day"=w628) -> (w634:T2)
        n275 = Generate User Event(user event=w626, event data cluster=TRUE ("event data")) -> ()  [unwired: 2 in, 2 out]
      }
      event "threshold cases": Value Change {
        n276 = event-data() -> ()  [unwired: 1 in, 6 out]
        n277 = local read "Country"() -> (w656:u16)
        n278 = property on="Country" class="Ring (strict)"("Val(Sgnl)"=w656) -> ()  [unwired: 2 in, 2 out]
      }
      event "Curve fit all data": Value Change {
        n279 = event-data() -> ("OldVal"=w659:bool)  [unwired: 1 in, 5 out]
        n280 = local write "Curve fit cursors"(w659) -> ()
        n281 = property on="calculate" class="Bool (strict)"("Val(Sgnl)"=TRUE ("Value (Signaling)")) -> ()  [unwired: 2 in, 2 out]
      }
      event "Curve fit cursors": Value Change {
        n282 = event-data() -> ("OldVal"=w662:bool)  [unwired: 1 in, 5 out]
        n283 = local write "Curve fit all data"(w662) -> ()
        n284 = property on="calculate" class="Bool (strict)"("Val(Sgnl)"=TRUE ("Value (Signaling)")) -> ()  [unwired: 2 in, 2 out]
      }
      event "XY Graph": Cursor Release {
        n285 = event-data() -> ("CursIdx"=w670:i32, "CursLoc"=w672:cluster{"X":dbl, "Y":dbl})  [unwired: 1 in, 7 out]
        n286 = Unbundle By Name(w665) -> ("country 1.first case date"=w664:timestamp)
        n287 = Unbundle By Name(w672) -> ("X"=w666:dbl)
        n288 = property on="relative graph" class="XYGraph (strict)"() -> ("CrsrList"=w671:T7)  [unwired: 2 in, 2 out]
        n289 = local read "Curve fit cursors"() -> (w674:bool)
        n290 = Equal?(x=w670, y=0) -> (x = y?=w679:bool)
        n291 = Equal?(x=w670, y=1) -> (x = y?=w678:bool)
        n292 = call "time to day.vi"("time offset"=w664, "time in seconds"=w666) -> ("fractional day"=w663:dbl)  [unwired: 1 out]
        n293 = Index Array(array=w671, index=w670) -> (element=w668:T8)
        n294 = Or(x=w679, y=w678) -> (x .or. y?=w673:bool)
        n295 = Bundle By Name(cluster=w668, "Position.X"=w663) -> (w667:T8)
        n296 = And(x=w673, y=w674) -> (x .and. y?=w675:bool)
        n297 = case shown="True" w675 {
          frame False {
          }
          frame True {
            n298 = property on="calculate" class="Bool (strict)"("Val(Sgnl)"=TRUE ("Value (Signaling)")) -> ()  [unwired: 2 in, 2 out]
          }
        }
        n299 = Replace Array Subset(array=w671, new element=w667, index=w670) -> (w669:T7)
        n300 = property on="relative graph" class="XYGraph (strict)"("CrsrList"=w669) -> ()  [unwired: 2 in, 2 out]
      }
      event "relative graph": Cursor Release {
        n301 = event-data() -> ("CursIdx"=w688:i32, "CursLoc"=w690:cluster{"X":dbl, "Y":dbl})  [unwired: 1 in, 7 out]
        n302 = Unbundle By Name(w684) -> ("country 1.first case date"=w682:timestamp)
        n303 = Unbundle By Name(w690) -> ("X"=w683:dbl)
        n304 = local read "Curve fit cursors"() -> (w692:bool)
        n305 = Equal?(x=w688, y=0) -> (x = y?=w697:bool)
        n306 = Equal?(x=w688, y=1) -> (x = y?=w696:bool)
        n307 = property on="XY Graph" class="XYGraph (strict)"() -> ("CrsrList"=w689:T7)  [unwired: 2 in, 2 out]
        n308 = call "day to time.vi"("Time offset"=w682, "day"=w683) -> ("day in seconds"=w681:dbl)  [unwired: 1 out]
        n309 = Index Array(array=w689, index=w688) -> (element=w686:T8)
        n310 = Or(x=w697, y=w696) -> (x .or. y?=w691:bool)
        n311 = And(x=w691, y=w692) -> (x .and. y?=w693:bool)
        n312 = Bundle By Name(cluster=w686, "Position.X"=w681) -> (w685:T8)
        n313 = case shown="True" w693 {
          frame False {
          }
          frame True {
            n314 = property on="calculate" class="Bool (strict)"("Val(Sgnl)"=TRUE ("Value (Signaling)")) -> ()  [unwired: 2 in, 2 out]
          }
        }
        n315 = Replace Array Subset(array=w689, new element=w685, index=w688) -> (w687:T7)
        n316 = property on="XY Graph" class="XYGraph (strict)"("CrsrList"=w687) -> ()  [unwired: 2 in, 2 out]
      }
      event "XY Graph": Scale Range Change {
        n317 = event-data() -> ("Kind"=w702:enum16{"X-Scale", "Y-Scale", "Z-Scale"}, "NewRange"=w701:T14)  [unwired: 1 in, 6 out]
        n318 = Unbundle By Name(w700) -> ("country 1.first case date"=w699:timestamp)
        n319 = case shown="\"Y-Scale\"" w702 {
          tunnel: w701 -> [w708 w712]
          tunnel: w699 -> [w703 _]
          frame "X-Scale", Default {
            n320 = Unbundle By Name(w708) -> ("Maximum"=w707:dbl, "Minimum"=w704:dbl)
            n321 = property on="calculate" class="Bool (strict)"("Val(Sgnl)"=TRUE ("Value (Signaling)")) -> ()  [unwired: 2 in, 2 out]
            n322 = call "time to day.vi"("time offset"=w703, "time in seconds"=w707) -> ("fractional day"=w706:dbl)  [unwired: 1 out]
            n323 = call "time to day.vi"("time offset"=w703, "time in seconds"=w704) -> ("fractional day"=w705:dbl)  [unwired: 1 out]
            n324 = property on="relative graph" class="XYGraph (strict)"("XScale.Maximum"=w706, "XScale.Minimum"=w705) -> ()  [unwired: 2 in, 2 out]
          }
          frame "Y-Scale" {
            n325 = Unbundle By Name(w712) -> ("Maximum"=w711:dbl, "Minimum"=w710:dbl)
            n326 = property on="relative graph" class="XYGraph (strict)"("YScale.Maximum"=w711, "YScale.Minimum"=w710) -> ()  [unwired: 2 in, 2 out]
          }
        }
      }
      event "relative graph": Scale Range Change {
        n327 = event-data() -> ("Kind"=w716:enum16{"X-Scale", "Y-Scale", "Z-Scale"}, "NewRange"=w715:T14)  [unwired: 1 in, 6 out]
        n328 = Unbundle By Name(w714) -> ("country 1.first case date"=w713:timestamp)
        n329 = case shown="\"Y-Scale\"" w716 {
          tunnel: w715 -> [w722 w724]
          tunnel: w713 -> [w717 _]
          frame "X-Scale", Default {
            n330 = Unbundle By Name(w722) -> ("Maximum"=w721:dbl, "Minimum"=w719:dbl)
            n331 = property on="calculate" class="Bool (strict)"("Val(Sgnl)"=TRUE ("Value (Signaling)")) -> ()  [unwired: 2 in, 2 out]
            n332 = call "day to time.vi"("Time offset"=w717, "day"=w721) -> ("day in seconds"=w720:dbl)  [unwired: 1 out]
            n333 = call "day to time.vi"("Time offset"=w717, "day"=w719) -> ("day in seconds"=w718:dbl)  [unwired: 1 out]
            n334 = property on="XY Graph" class="XYGraph (strict)"("XScale.Maximum"=w720, "XScale.Minimum"=w718) -> ()  [unwired: 2 in, 2 out]
          }
          frame "Y-Scale" {
            n335 = Unbundle By Name(w724) -> ("Maximum"=w726:dbl, "Minimum"=w725:dbl)
            n336 = property on="XY Graph" class="XYGraph (strict)"("YScale.Maximum"=w726, "YScale.Minimum"=w725) -> ()  [unwired: 2 in, 2 out]
          }
        }
      }
      event "Data": Value Change {
        n337 = event-data() -> ()  [unwired: 1 in, 6 out]
        n338 = property on="calculate" class="Bool (strict)"("Val(Sgnl)"=TRUE ("Value (Signaling)")) -> ()  [unwired: 2 in, 2 out]
      }
      event "X-axis absolute": Value Change {
        n339 = event-data() -> ("OldVal"=w734:bool, "NewVal"=w731:bool)  [unwired: 1 in, 4 out]
        n340 = local write "X-axis relative"(w734) -> ()
        n341 = Select(t=enum32{"Absolute", "Relative"}."Absolute" ("abs or rel"), s=w731, f=enum32{"Absolute", "Relative"}."Relative") -> (s? t:f=w729:enum32{"Absolute", "Relative"})
        n342 = local write "abs or rel"(w729) -> ()
        n343 = property on="calculate" class="Bool (strict)"("Val(Sgnl)"=TRUE ("Value (Signaling)")) -> ()  [unwired: 2 in, 2 out]
      }
      event "X-axis relative": Value Change {
        n344 = event-data() -> ("OldVal"=w741:bool, "NewVal"=w736:bool)  [unwired: 1 in, 4 out]
        n345 = local write "X-axis absolute"(w741) -> ()
        n346 = property on="calculate" class="Bool (strict)"("Val(Sgnl)"=TRUE ("Value (Signaling)")) -> ()  [unwired: 2 in, 2 out]
        n347 = Select(t=enum32{"Absolute", "Relative"}."Relative" ("abs or rel"), s=w736, f=enum32{"Absolute", "Relative"}."Absolute") -> (s? t:f=w739:enum32{"Absolute", "Relative"})
        n348 = local write "abs or rel"(w739) -> ()
      }
      event "Y-axis normalised": Value Change {
        n349 = event-data() -> ("OldVal"=w744:bool)  [unwired: 1 in, 5 out]
        n350 = local write "Y-axis absolute"(w744) -> ()
        n351 = property on="calculate" class="Bool (strict)"("Val(Sgnl)"=TRUE ("Value (Signaling)")) -> ()  [unwired: 2 in, 2 out]
      }
      event "Y-axis absolute": Value Change {
        n352 = event-data() -> ("OldVal"=w747:bool)  [unwired: 1 in, 5 out]
        n353 = local write "Y-axis normalised"(w747) -> ()
        n354 = property on="calculate" class="Bool (strict)"("Val(Sgnl)"=TRUE ("Value (Signaling)")) -> ()  [unwired: 2 in, 2 out]
      }
      event "Curve 1", "Curve 2": Value Change {
        n355 = event-data() -> ()  [unwired: 1 in, 6 out]
        n356 = property on="calculate" class="Bool (strict)"("Val(Sgnl)"=TRUE ("Value (Signaling)")) -> ()  [unwired: 2 in, 2 out]
        n357 = Unbundle By Name(w751) -> ("Update plot names"=w750:refnum<user-event>)
        n358 = Generate User Event(user event=w750, event data cluster=TRUE ("event data")) -> ()  [unwired: 2 in, 2 out]
      }
      event "Presets": Value Change {
        n359 = event-data() -> ("NewVal"=w759:bool)  [unwired: 1 in, 5 out]
        n360 = case shown="True" w759 {
          tunnel: w758 -> [w761 w768]
          tunnel: [w761 w765] -> w757
          tunnel: w756 -> [_ w767]
          tunnel: w755 -> [_ w766]
          tunnel: w754 -> [_ w763]
          tunnel: w753 -> [_ w762]
          frame False {
          }
          frame True {
            n361 = local read "Curve fit all data"() -> (w777:bool)
            n362 = property on="XY Graph" class="XYGraph (strict)"() -> ("CrsrList"=w773:T7)  [unwired: 2 in, 2 out]
            n363 = local read "X-axis absolute"() -> (w774:bool)
            n364 = property on="Country" class="Ring (strict)"() -> ("Strings []"=w782:string[])  [unwired: 2 in, 2 out]
            n365 = Index Array(array=w773) -> (element #1=w772:T8, element #2=w771:T8)  [unwired: 2 in]
            n366 = local read "threshold cases"() -> (w764:u32)
            n367 = local read "Curve 1"() -> (w776:enum16{"Exponential", "Logarithm", "No curve"})
            n368 = local read "Curve 2"() -> (w775:enum16{"Exponential", "Logarithm", "No curve"})
            n369 = local read "Compare with"() -> (w783:u16)
            n370 = Unbundle By Name(w772) -> ("Position.X"=w770:dbl)
            n371 = Unbundle By Name(w771) -> ("Position.X"=w769:dbl)
            n372 = local read "Data"() -> (w778:u16)
            n373 = local read "Country"() -> (w784:u16)
            n374 = Bundle By Name(cluster=T6 {"Country 1 index"=201, "Country 2 index"=0, "countries"=[], "Data"=0, "Curve fit all data"=TRUE, "Curve 1 type"=enum."Exponential", "Curve 2 type"=enum."Exponential", "absolute?"=TRUE, "cursor 1 "=0.0, "cursor 2 "=0.0, "threshold cases"=50}, "Country 1 index"=w784, "Country 2 index"=w783, "countries"=w782, "Data"=w778, "Curve fit all data"=w777, "Curve 1 type"=w776, "Curve 2 type"=w775, "absolute?"=w774, "cursor 1"=w770, "cursor 2"=w769, "threshold cases"=w764) -> (w781:T6)
            n375 = call "presets dialog.vi"("Cluster in"=w781) -> ("Load?"=w780:bool, "Cluster out"=w779:T6)  [unwired: 9 in]
            n376 = case shown="True" w780 {
              tunnel: w779 -> [_ w795]
              tunnel: w768 -> [w786 w791]
              tunnel: w767 -> [_ w794]
              tunnel: w766 -> [_ w793]
              tunnel: [w786 w792] -> w765
              tunnel: w763 -> [_ w788]
              tunnel: w762 -> [_ w787]
              frame False {
              }
              frame True {
                n377 = stacked-sequence {
                  seq-local: [_ w829 _ _] -> [_ _ w840 w852]
                  seq-local: [w801 _ _ _] -> [_ _ w839 _]
                  seq-local: [w800 _ _ _] -> [_ _ w831 _]
                  tunnel: w795 -> [w816 _ _ _]
                  tunnel: w791 -> [_ w828 _ _]
                  tunnel: w794 -> [_ w822 _ w854]
                  tunnel: w793 -> [_ w821 _ w853]
                  tunnel: [_ _ _ w851] -> w792
                  tunnel: w788 -> [_ w818 _ w846]
                  tunnel: w787 -> [_ w817 _ w845]
                  frame #0 {
                    n378 = property on="XY Graph" class="XYGraph (strict)"() -> ("CrsrList"=w802:T7)  [unwired: 2 in, 2 out]
                    n379 = Unbundle By Name(w816) -> ("Data"=w815:u16, "Country 1 index"=w814:i32, "Country 2 index"=w813:i32, "Curve fit all data"=w811:bool, "Curve 1 type"=w810:enum16{"Exponential", "Logarithm", "No curve"}, "Curve 2 type"=w809:enum16{"Exponential", "Logarithm", "No curve"}, "absolute?"=w799:bool, "cursor 1"=w801:dbl, "cursor 2"=w800:dbl)
                    n380 = Index Array(array=w802) -> (element #1=w803:T8, element #2=w804:T8)  [unwired: 2 in]
                    n381 = Bundle By Name(cluster=w803, "Position.X"=w801) -> (w805:T8)
                    n382 = Bundle By Name(cluster=w804, "Position.X"=w800) -> (w806:T8)
                    n383 = Not(x=w811) -> (.not. x?=w812:bool)
                    n384 = Not(x=w799) -> (.not. x?=w808:bool)
                    n385 = Select(t=enum32{"Absolute", "Relative"}."Absolute" ("abs or rel"), s=w799, f=enum32{"Absolute", "Relative"}."Relative") -> (s? t:f=w797:enum32{"Absolute", "Relative"})
                    n386 = local write "Data"(w815) -> ()
                    n387 = local write "Country"(w814) -> ()
                    n388 = local write "Compare with"(w813) -> ()
                    n389 = local write "Curve fit all data"(w811) -> ()
                    n390 = local write "Curve fit cursors"(w812) -> ()
                    n391 = local write "Curve 1"(w810) -> ()
                    n392 = local write "Curve 2"(w809) -> ()
                    n393 = local write "X-axis absolute"(w799) -> ()
                    n394 = local write "X-axis relative"(w808) -> ()
                    n395 = local write "abs or rel"(w797) -> ()
                    n396 = Build Array(w805, w806) -> (w807:T13)
                    n397 = property on="XY Graph" class="XYGraph (strict)"("CrsrList"=w807) -> ()  [unwired: 2 in, 2 out]
                  }
                  frame #1 {
                    n398 = local read "threshold cases"() -> (w823:u32)
                    n399 = local read "Country"() -> (w819:u16)
                    n400 = call "parse CSV files.vi"("threshold cases"=w823, "SA data"=w817, "US data"=w818, "deaths CSV"=w821, "country index"=w819, "cases CSV"=w822) -> ("new deaths per day"=w820:i32[], "days"=w825:i32[], "new cases per day"=w826:i32[], "first case date"=w827:timestamp, "cumulative cases"=w824:i32[], "cumulative deaths"=w830:i32[])
                    n401 = Bundle By Name(cluster=w828, "country 1.new cases per day"=w826, "country 1.days"=w825, "country 1.cumulative cases"=w824, "country 1.first case date"=w827, "country 1.deaths"=w830, "country 1.new deaths per day"=w820) -> (w829:T2)
                  }
                  frame #2 {
                    n402 = Unbundle By Name(w840) -> ("country 1.first case date"=w837:timestamp)
                    n403 = property on="relative graph" class="XYGraph (strict)"() -> ("CrsrList"=w844:T7)  [unwired: 2 in, 2 out]
                    n404 = call "time to day.vi"("time offset"=w837, "time in seconds"=w839) -> ("fractional day"=w841:dbl)  [unwired: 1 out]
                    n405 = call "time to day.vi"("time offset"=w837, "time in seconds"=w831) -> ("fractional day"=w833:dbl)  [unwired: 1 out]
                    n406 = Index Array(array=w844) -> (element #1=w842:T8, element #2=w832:T8)  [unwired: 2 in]
                    n407 = Bundle By Name(cluster=w842, "Position.X"=w841) -> (w838:T8)
                    n408 = Bundle By Name(cluster=w832, "Position.X"=w833) -> (w834:T8)
                    n409 = Replace Array Subset(array=w844, new element #1=w838, index #1=0, new element #2=w834, index #2=1 ("index")) -> (w843:T7)
                    n410 = property on="relative graph" class="XYGraph (strict)"("CrsrList"=w843) -> ()  [unwired: 2 in, 2 out]
                  }
                  frame #3 {
                    n411 = local read "Compare with"() -> (w850:u16)
                    n412 = local read "threshold cases"() -> (w855:u32)
                    n413 = Greater Than 0?(x=w850) -> (x > 0?=w849:bool)
                    n414 = case shown="True" w849 {
                      tunnel: [w861 w875] -> w860
                      tunnel: [timestamp(0 s since 1904-01-01) ("first case date") w874] -> w859
                      tunnel: [w861 w873] -> w858
                      tunnel: [w861 w872] -> w857
                      tunnel: [w861 w871] -> w856
                      tunnel: w855 -> [_ w870]
                      tunnel: w854 -> [_ w869]
                      tunnel: w853 -> [_ w868]
                      tunnel: w850 -> [_ w867]
                      tunnel: [w861 w866] -> w847
                      tunnel: w846 -> [_ w864]
                      tunnel: w845 -> [_ w863]
                      frame False {
                        w861 = i32[] [] ("new cases per day")
                      }
                      frame True {
                        n415 = Decrement(x=w867) -> (x-1=w865:u16)
                        n416 = call "parse CSV files.vi"("threshold cases"=w870, "SA data"=w863, "US data"=w864, "deaths CSV"=w868, "country index"=w865, "cases CSV"=w869) -> ("new deaths per day"=w866:i32[], "days"=w872:i32[], "new cases per day"=w873:i32[], "first case date"=w874:timestamp, "cumulative cases"=w871:i32[], "cumulative deaths"=w875:i32[])
                      }
                    }
                    n417 = Bundle By Name(cluster=w852, "country 2.new cases per day"=w858, "country 2.days"=w857, "country 2.cumulative cases"=w856, "country 2.first case date"=w859, "country 2.deaths"=w860, "country 2.new deaths per day"=w847) -> (w851:T2)
                    n418 = property on="calculate" class="Bool (strict)"("Val(Sgnl)"=TRUE ("Value (Signaling)")) -> ()  [unwired: 2 in, 2 out]
                  }
                }
                n419 = Unbundle By Name(w791) -> ("Update plot names"=w790:refnum<user-event>)
                n420 = Generate User Event(user event=w790, event data cluster=TRUE ("event data")) -> ()  [unwired: 2 in, 2 out]
              }
            }
          }
        }
        n421 = local write "Presets"(FALSE ("Presets")) -> ()
      }
      event "compare": Value Change {
        n422 = event-data() -> ()  [unwired: 1 in, 6 out]
        n423 = call "compare multiple countries window.vi"("Aggregate indexes"=w877, "Countries"=w878, "SA data"=w876, "US data"=w879, "Populations"=w880, "deaths CSV"=w882, "cases CSV"=w883) -> ()  [unwired: 5 in]
        n424 = local write "compare"(FALSE ("compare")) -> ()
      }
      event "sorted": Value Change {
        n425 = event-data() -> ()  [unwired: 1 in, 6 out]
        n426 = call "compare top countries window.vi"("SA data"=w885, "Countries"=w887, "Aggregate indexes"=w886, "Populations"=w889, "US data"=w888, "deaths CSV"=w891, "cases CSV"=w892) -> ()  [unwired: 5 in]
        n427 = local write "sorted"(FALSE ("compare")) -> ()
      }
      event "Moving average": Value Change {
        n428 = event-data() -> ("NewVal"=w899:bool)  [unwired: 1 in, 5 out]
        n429 = Select(t=T1."Enabled" ("Disabled"), s=w899, f=T1."Disabled and Grayed Out" ("Disabled")) -> (s? t:f=w896:T1)
        n430 = property on="Days" class="DigNum (strict)"("DisabledEnum"=w896) -> ()  [unwired: 2 in, 2 out]
        n431 = property on="calculate" class="Bool (strict)"("Val(Sgnl)"=TRUE ("Value (Signaling)")) -> ()  [unwired: 2 in, 2 out]
      }
      event "Days": Value Change {
        n432 = event-data() -> ()  [unwired: 1 in, 6 out]
        n433 = property on="calculate" class="Bool (strict)"("Val(Sgnl)"=TRUE ("Value (Signaling)")) -> ()  [unwired: 2 in, 2 out]
      }
      event User Event {
        n434 = event-data() -> ()  [unwired: 1 in, 5 out]
        n435 = property on="Compare with" class="Ring (strict)"() -> ("Strings []"=w916:string[], "Value"=w911:u16)  [unwired: 2 in, 2 out]
        n436 = property on="Country" class="Ring (strict)"() -> ("Strings []"=w918:string[], "Value"=w917:u16)  [unwired: 2 in, 2 out]
        n437 = local read "Curve 1"() -> (w914:enum16{"Exponential", "Logarithm", "No curve"})
        n438 = Greater Than 0?(x=w911) -> (x > 0?=w910:bool)
        n439 = Equal?(x=enum16{"Exponential", "Logarithm", "No curve"}."No curve" ("Curve 1"), y=w914) -> (x = y?=w913:bool)
        n440 = Index Array(array=w918, index=w917) -> (element=w912:string)
        n441 = Index Array(array=w916, index=w911) -> (element=w908:string)
        n442 = case shown="False" w913 {
          tunnel: w912 -> [w938 w941]
          tunnel: [w936 w940] -> w909
          frame False {
            n443 = Concatenate Strings(w938, "- curve") -> (w937:string)
            n444 = Build Array(w937, w938) -> (w936:string[])
          }
          frame True {
            n445 = Build Array(w941) -> (w940:string[])
          }
        }
        n446 = local read "Curve 2"() -> (w905:enum16{"Exponential", "Logarithm", "No curve"})
        n447 = case shown="True" w910 {
          tunnel: w909 -> [w920 w922]
          tunnel: w908 -> [_ w923]
          tunnel: [w920 w921] -> w907
          tunnel: enum16{"Exponential", "Logarithm", "No curve"}."No curve" ("y") -> [_ w926]
          tunnel: w905 -> [_ w925]
          frame False {
          }
          frame True {
            n448 = Equal?(x=w925, y=w926) -> (x = y?=w924:bool)
            n449 = case shown="False" w924 {
              tunnel: w923 -> [w927 w934]
              tunnel: w922 -> [w930 w935]
              tunnel: [w929 w933] -> w921
              frame False {
                n450 = Concatenate Strings(w927, "- curve") -> (w932:string)
                n451 = Build Array(w932, w927) -> (w928:string[])
                n452 = Build Array (concatenate)(w930, w928) -> (w929:string[])
              }
              frame True {
                n453 = Build Array (concatenate)(w935, w934) -> (w933:string[])
              }
            }
          }
        }
        n454 = for {
          tunnel: w907 -> [w945] mode=indexing
          tunnel: [w944] -> w904
          i -> [w946]
          n455 = property on="relative graph" class="XYGraph (strict)"("Active Plot"=w946) -> (error out=w942:errorcluster)  [unwired: 2 in, 1 out]
          n456 = property on="XY Graph" class="XYGraph (strict)"("Active Plot"=w946) -> (error out=w943:errorcluster)  [unwired: 2 in, 1 out]
          n457 = property on="relative graph" class="XYGraph (strict)"(error in=w942, "Plot.Plot Name"=w945) -> ()  [unwired: 1 in, 2 out]
          n458 = property on="XY Graph" class="XYGraph (strict)"(error in=w943, "Plot.Plot Name"=w945) -> (error out=w944:errorcluster)  [unwired: 1 in, 1 out]
        }
        n459 = invoke on="XY Graph" class="XYGraph (strict)" method="FitControlToPane"(error in=w904) -> (error out=w903:errorcluster)  [unwired: 2 in, 2 out]
        n460 = invoke on="relative graph" class="XYGraph (strict)" method="FitControlToPane"(error in=w903) -> ()  [unwired: 2 in, 3 out]
      }
    }
  }
  n461 = global read "Globals.vi" "version"() -> (→"Version":u32)
  n462 = Unbundle By Name(w7) -> ("Update plot names"=w6:refnum<user-event>)
  n463 = Unregister For Events(event registration refnum=w5) -> (error out=w4:errorcluster)  [unwired: 1 in]
  n464 = Destroy User Event(user event=w6, error in=w4) -> ()  [unwired: 1 out]
